vi "plcHMI_rev6.vi"() -> ()   [LabVIEW 2020]
doc: "ADS continuos synchronous write example using base blocks. \n\nThe client writes data synchronously and does wait for the respose from server."
uses:
  Agilent/AgilentTotalCluster.ctl
  Agilent/AgilentControl.ctl
  Agilent/Channel Config.ctl
  <vilib>/Platform/TimedLoop/XDataNode/timing_clust.ctl
  <vilib>/Platform/TimedLoop/XDataNode/nitl_modes.ctl
  <vilib>/Platform/TimedLoop/XDataNode/wakeup.ctl
  <userlib>/Beckhoff-LabVIEW-Interface/_DependsOn/With TypeResolving/Write Sync Single TypeResolved.vi
  <userlib>/Beckhoff-LabVIEW-Interface/_DependsOn/With TypeResolving/Read Sync Single TypeResolved.vi
  <vilib>/Platform/TimedLoop/XDataNode/XDataNode.xnode
  <vilib>/Platform/TimedLoop/XDataNode/XDNodeRunTimeDep.lvlib
panel:
  in  "Tab Control":T1(tab)
  out "error out":errorcluster
  in  "Symbol file path - MUST BE ENTERED\nLoad \"ADS Write AND Read Symbols REV X.X.xml\"":path
  out "bHasMached":bool
  out "Write Status":bool
  out "Read Status":bool
  in  "EXIT HMI":bool caption="STOP HMI\nEXIT HMI"
  out "Internal TwinCAT Handle ID Maps":dbl format="%#_12g"
  in  "802L TDK PSU Voltage Rating (abs(Volts))":i32=12000 min=1 max=50000
  in  "802L TDL PSU Peak Power (J/s)":i32=9000 min=1 max=50000
  in  "HVPS Model":u16(ring) items=["802L-12kV,9000J/s", "802L+50kV,9000J/s", "Other"]
  out "Test Interval Fault":bool
  in  "Cycle Time (Sec)":i32=15 min=0
  in  "Voltage Held by PSU":bool
  in  "Log Capacitor Voltage":bool
  in  "Log Temperature Data":bool
  out "Time Since Last Shot":string caption="Elapsed Time Text"
  in  "Duty Cycle":dbl
  in  "Current Control":bool
  out "Expected Voltage":i16
  in  "Dump":bool
  out "EOC":bool
  out "Maximum Test Number Reached":bool
  out "SCR Ready":bool
  in  "START":bool
  in  "STOP":bool
  in  "Hold":bool
  in  "Charge":bool
  in  "Shot":bool
  in  "HV Switch Mode":bool
  in  "CLEAR FAULT":bool
  in  "Manual/Auto":bool=TRUE
  out "Test Interval (Sec)":i32=15 min=0
  in  "Capacitance (uF)":sgl=1e-13 min=0 max=10000 format="%#_6f"
  in  "Target Charge Volt (V) - Min 1500V":i32 min=-12000 max=50000 step=1
  out "Estimated Charge Time (seconds)":sgl
  in  "Hold Time Before Shot (seconds)":sgl max=1000
  in  "Max Number of Shots (Test intervals)":i16=1 min=1
  out "Shot Number":i16
  out "Charge Fault":bool=TRUE
  out "Discharge Fault":bool=TRUE
  out "Hold Fault":bool=TRUE
  out "Cap 1 Temp\nExceeded Fault":bool=TRUE
  out "Ambient Temp\nExceeded Fault":bool=TRUE
  out "PSU Fault":bool=TRUE
  out "Control Sys Fault":bool=TRUE
  out "test Running":bool
  out "Test State":string
  out "Cap 1 Voltage":i16
  out "Cap 1 Temperature":i16
  in  "Capacitor Voltage Data Log File Path (.xlsx)":path
  out "Load Temperature":i16
  out "Soft Dump Temp":i16
  out "Ambient Temp":i16
  out "Waveform Chart - Capacitor Voltage (Probe, abs(Volts))":dbl(graph)
  in  "Manual Charge Time (seconds)":sgl max=90
  in  "Reset Test Number":bool
  in  "Cap 1 Fault Temp (Cel)":i16 min=0 max=300
  in  "Capacitor Temperature Data Log File Path (.xlsx)":path
  out "Cap 1 Voltage (HVPS)":i16
  in  "50kV PSU Charger Selected\n(OFF = 12kV Selected, ON = 50kV) Selected":bool
  in  "Cap Rated Voltage (V)":u16 max=50000
  out "Target Voltage Exceeded\nCap Rating Voltage":bool=TRUE
  in  "Soft Dump Temp Thres (Cel)":i16 min=0 max=500
  in  "Load Temp Thres (Cel)":i16 min=0 max=500
  in  "Ambient Temp Thres (Cel)":i16 min=0 max=500
  out "All Temp In Range":bool=TRUE
  out "Load Temp Fault":bool=TRUE
  out "Capacitor Voltage":cluster{dbl, dbl}(graph)
  out "EOC":i16(graph)
  out "Soft Exception":bool
  out "PSU HV FB Fault":bool
  out "Charge FB Fault":bool
  out "Softdump FB Fault":bool
  out "SCR FB":i16(graph)
  out "Spark Gap Voltage":i16(graph)
  in  "CH4 Vertical Units":string(combo)="V"
  in  "CH4 Vertical Units/div":dbl=2.0
  in  "Toggle Scope Scale":bool
  in  "CH1 Vertical Units/div":dbl=2.0
  in  "CH1 Vertical Units":string(combo)="V"
  in  "Horizontal Units":enum16{"us", "ms", "s"}(ring)
  in  "Horizontal Units/div":dbl=200.0
  out "Download":bool
  in  "Single":bool
  in  "Stop":bool
  out "Scope Trig":bool
  in  "Agilent Array":T2[](array[typedef])
  out "Process Step":u8
  out "Stop Loops":bool
  # "CONFIGURATION"
  # "Press STOP HMI instead of\nLabView Abort Execution"
  # "PSU V Rating, Peak Power\nactive when OTHER\nis selected"
  # "INPUT VARIABLES - For TDK Lambda 802L\nMust be written to before START"
  # "FAULT STATUSES"
  # "Set to -1 for automated\nfull charge to setpoint"
  # "MANUAL CONTROLS"
  # "Does not record during \"wait\" and appends to data file. Must be named with .xlsx"
  # "HV Switch Configuration"
  # "Records during \"Test Running.\" Must be named with .xlsx"
  # "Control Sys Faults"
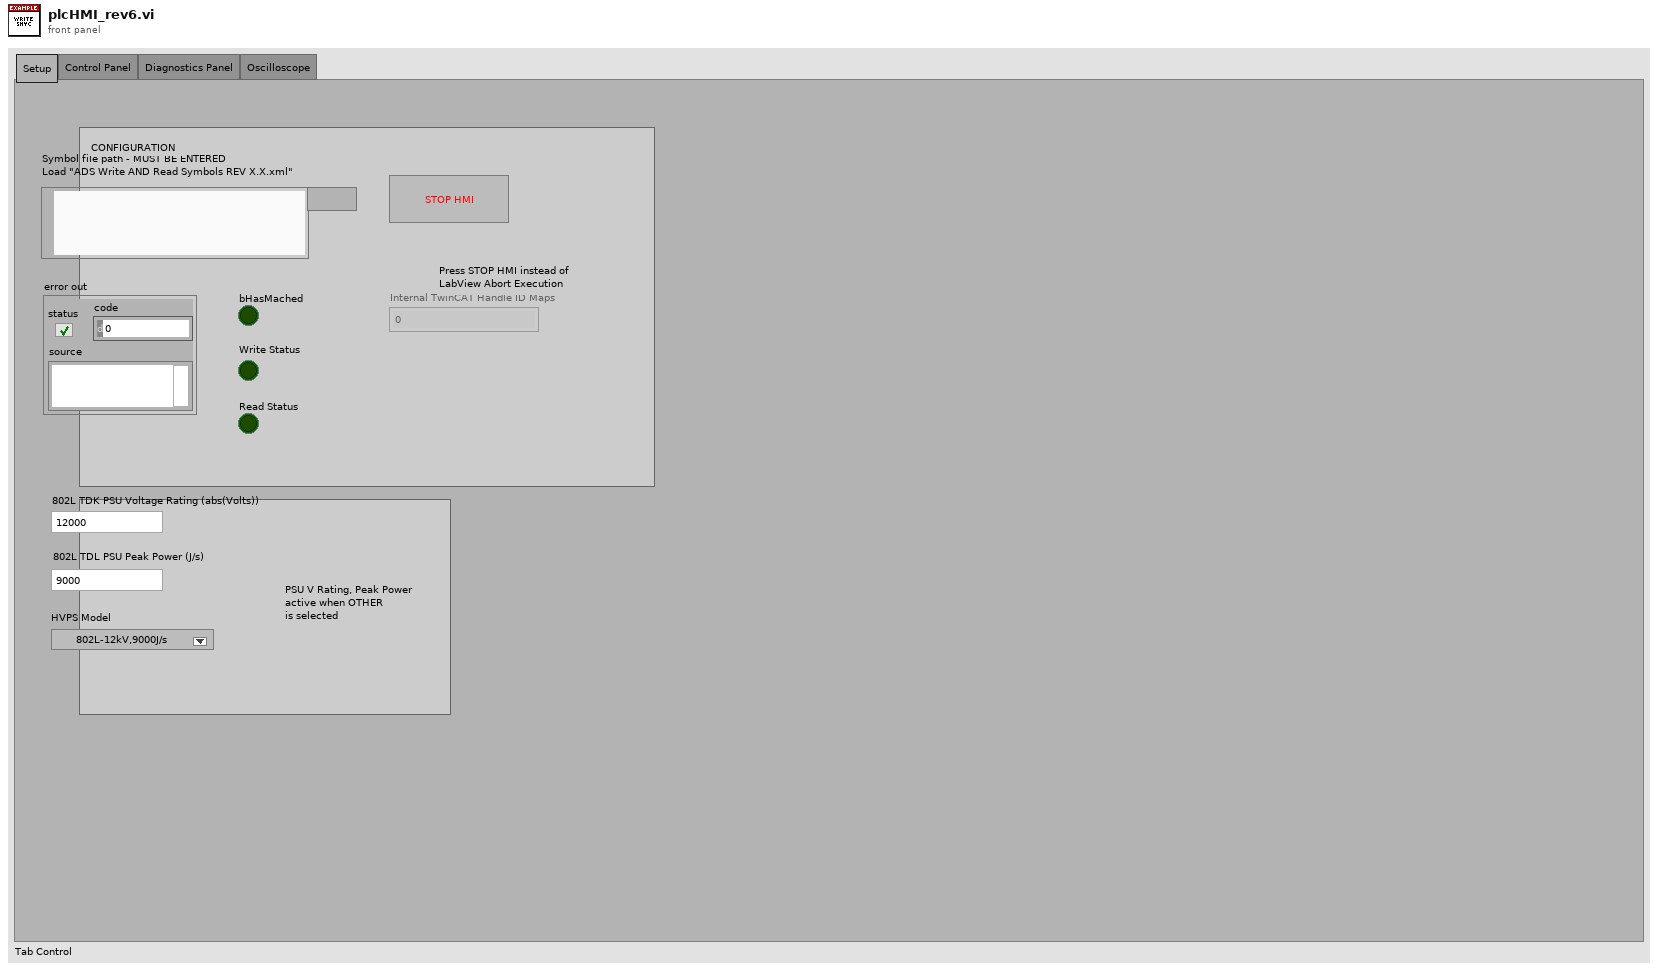
[diagram p1: front panel]
types:
  T1 = enum32{"Setup", "Control Panel", "Diagnostics Panel", "Oscilloscope"}
  T2 = typedef "AgilentTotalCluster.ctl" = cluster{"Agilent Graph":waveform(dbl)[], "Agilent Control":T3, "Agilent Setup Error":errorcluster, "Agilent Present":bool, "Enabled":bool}
  T3 = typedef "AgilentControl.ctl" = cluster{"Trig?":bool, "VISA session":refnum<visa-resource-name>, "Setup to Load":string, "Timeout (ms)":u32, "Desired Samp":enum32{"100", "250", "500", "1000", "2000", "5000", "10000", "20000", "50000", "100000", "200000", "500000", "1000000", "2000000", "4000000", "8000000"}, "Captured Samp":i32, "Desired Channels":T4[]}
  T4 = typedef "Channel Config.ctl" = cluster{"Chan Index":enum16{"Channel1", "Channel2", "Channel3", "Channel4", "MATH"}, "Name":string, "Samples":i32}
  T5 = typedef "XDNodeRunTimeDep.lvlib/timing_clust.ctl" = cluster{"Expected End [f-1]":u64, "Actual End [f-1]":u64, "Finished Late? [f-1]":bool, "Expected End [i-1]":u64, "Actual End [i-1]":u64, "Finished Late? [i-1]":bool, "Expected Start [i]":u64, "Actual Start [i]":u64, "Expected Start [f]":u64, "Actual Start [f]":u64, "Source Name":string, "Structure Name":string, "Period":i64, "Deadline":i64, "Offset":i64, "Start":i64, "Priority":i32, "Timeout":i32, "Mode":T6, "Wakeup Reason":T7, "Error":errorcluster, "Source Type":string, "Secondary Source Type":string, "Global End Time":u64, "Global Start Time":u64, "Frame Duration":u64, "Iteration Duration":u64, "Assigned CPU":i32, "I/O Scan Engine Mode":u32}
  T6 = typedef "XDNodeRunTimeDep.lvlib/nitl_modes.ctl" = enum32{"No Change", "Process missed periods, maintain original phase", "Discard missed periods, maintain original phase", "Process missed periods, ignore original phase", "Discard missed periods, ignore original phase"}
  T7 = typedef "XDNodeRunTimeDep.lvlib/wakeup.ctl" = enum32{"Normal", "Aborted", "Asynchronous wakeup", "Timing source error", "Timed loop error", "Timeout"}
  T8 = cluster{"Agilent Array[0]":T2, "Agilent Array[1]":T2, "Agilent Array[2]":T2, "Agilent Array[3]":T2, "Agilent Array[4]":T2, "Agilent Array[5]":T2, "Agilent Array[6]":T2, "Agilent Array[7]":T2, "Agilent Array[8]":T2}
  T9 = enum32{"100", "250", "500", "1000", "2000", "5000", "10000", "20000", "50000", "100000", "200000", "500000", "1000000", "2000000", "4000000", "8000000"}
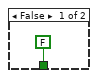
[diagram p2: hidden frame]
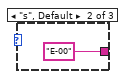
[diagram p5: hidden frame]
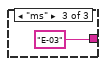
[diagram p6: hidden frame]
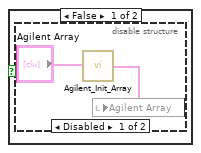
[diagram p7: hidden frame]
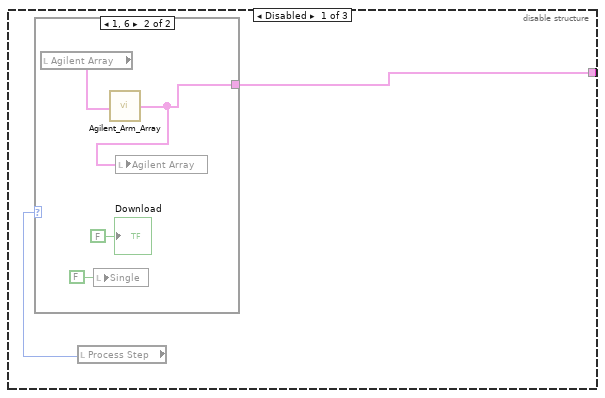
[diagram p11: hidden frame]
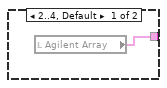
[diagram p12: hidden frame]
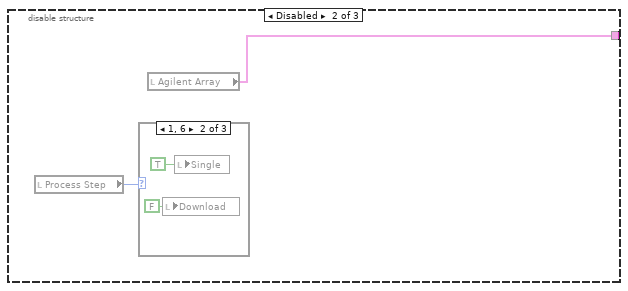
[diagram p13: hidden frame]
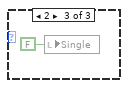
[diagram p15: hidden frame]
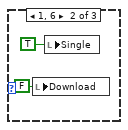
[diagram p17: hidden frame]
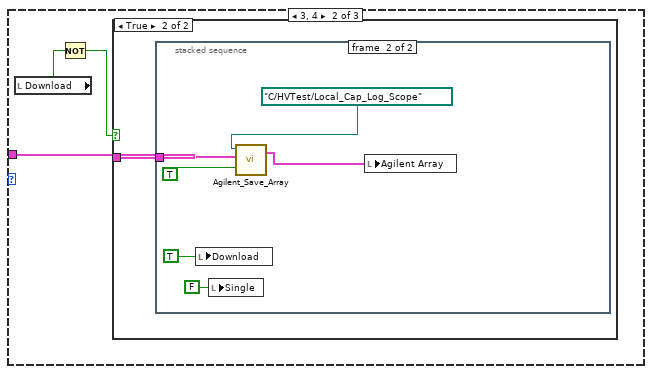
[diagram p19: hidden frame]
diagram:
  w115 = u16 17 items=["SyncLatest"=17, "AsyncLatest"=33] ("WriterMode")
  w185 = u16 33 items=["SyncLatest"=17, "AsyncLatest"=33] ("WriterMode")
  w225 = u16 33 items=["SyncLatest"=17, "AsyncLatest"=33] ("WriterMode")
  w244 = u16 33 items=["SyncLatest"=17, "AsyncLatest"=33] ("WriterMode")
  w263 = u16 33 items=["SyncLatest"=17, "AsyncLatest"=33] ("WriterMode")
  w282 = u16 33 items=["SyncLatest"=17, "AsyncLatest"=33] ("WriterMode")
  w301 = u16 33 items=["SyncLatest"=17, "AsyncLatest"=33] ("WriterMode")
  w320 = u16 17 items=["SyncLatest"=17, "AsyncLatest"=33] ("WriterMode")
  w339 = u16 17 items=["SyncLatest"=17, "AsyncLatest"=33] ("WriterMode")
  w358 = u16 17 items=["SyncLatest"=17, "AsyncLatest"=33] ("WriterMode")
  w377 = u16 17 items=["SyncLatest"=17, "AsyncLatest"=33] ("WriterMode")
  w396 = u16 17 items=["SyncLatest"=17, "AsyncLatest"=33] ("WriterMode")
  w415 = u16 17 items=["SyncLatest"=17, "AsyncLatest"=33] ("WriterMode")
  w434 = u16 17 items=["SyncLatest"=17, "AsyncLatest"=33] ("WriterMode")
  w449 = u16 17 items=["SyncLatest"=17, "AsyncLatest"=33] ("WriterMode")
  # "Variables/ Control"
  # "Documentation:\nCode separated vertically into two main sections - Write and read\nThey are further separated into BOOL and numeric\nThe OR gates wire all the error lines and the EXIT HMI button to a WHILE LOOP STOP\nThere current delay time on the routine is 100ms\nAll the AND gates connect the typecast resolve lines to the bHasMatched indicator\nThe second and third set of AND gates connect the write statuses to the Write Status indicator\nThe same is done for the read status indicator"
  # "WRITE NUMERICS"
  # "WRITE BOOLS"
  # "Select Symbol N"
  # "Read Initialization"
  # "Release \nTypeResolver"
  # "Release Writer"
  # "Send Request"
  # "Init \nTypeResolver"
  # "Init Writer"
  # "Select Symbol"
  # "Initialization"
  # "Call Release handle block\nat the end, when all nodes\nhave finished their execution"
  # "There must be only one release\nafter every init block.\nRelease block must be called\nalways at the end."
  # "Release"
  # "Symbol Interface"
  n1 = disable-structure shown="Enabled" {
    disable-tunnel: [w455 _] -> w453
    disable-tunnel: [w454 w457] -> w452
    frame Disabled {
      # "Using Symbol Interface"
      n2 = call <userlib>:"Symbol Interface.vi"() -> ("PortInfo"=w454:string, "error out"=w455:errorcluster)  [unwired: 14 in]
    }
    frame Enabled {
      # "Using Symbol File"
      n3 = Path To String(path="Symbol file path - MUST BE ENTERED\nLoad \"ADS Write AND Read Symbols REV X.X.xml\"") -> (string=w457:string)
    }
  }
  n4 = call <userlib>:"Init.vi"("XMLDescription"=w452, "error in (no error)"=w453) -> ("Handle"=w65:u32, "ReadGrpSymbols"=w5:string[], "WriteGrpSymbols"=w10:string[], "error out"=w32:errorcluster)  [unwired: 9 in, 1 out]
  n5 = Index Array(array=w10, index=0) -> (element=w43:string)
  n6 = Index Array(array=w10, index=26) -> (element=w9:string)
  n7 = Index Array(array=w10, index=24) -> (element=w16:string)
  n8 = Index Array(array=w10, index=23) -> (element=w22:string)
  n9 = Index Array(array=w10, index=22) -> (element=w25:string)
  n10 = Index Array(array=w10, index=25) -> (element=w13:string)
  n11 = Index Array(array=w10, index=21) -> (element=w53:string)
  n12 = Index Array(array=w10, index=20) -> (element=w58:string)
  n13 = Index Array(array=w10, index=14) -> (element=w33:string)
  n14 = Index Array(array=w10, index=9) -> (element=w302:string)
  n15 = Index Array(array=w10, index=10) -> (element=w283:string)
  n16 = Index Array(array=w10, index=12) -> (element=w245:string)
  n17 = Index Array(array=w10, index=11) -> (element=w264:string)
  n18 = Index Array(array=w10, index=13) -> (element=w226:string)
  n19 = Index Array(array=w10, index=18) -> (element=w66:string)
  n20 = Index Array(array=w10, index=19) -> (element=w59:string)
  n21 = Index Array(array=w10, index=7) -> (element=w321:string)
  n22 = Index Array(array=w10, index=2) -> (element=w416:string)
  n23 = Index Array(array=w10, index=3) -> (element=w397:string)
  n24 = Index Array(array=w10, index=5) -> (element=w359:string)
  n25 = Index Array(array=w10, index=4) -> (element=w378:string)
  n26 = Index Array(array=w10, index=6) -> (element=w340:string)
  n27 = Index Array(array=w10, index=1) -> (element=w435:string)
  n28 = Index Array(array=w10, index=16) -> (element=w36:string)
  n29 = Index Array(array=w10, index=8) -> (element=w114:string)
  n30 = Index Array(array=w10, index=15) -> (element=w186:string)
  n31 = Index Array(array=w10, index=17) -> (element=w38:string)
  n32 = call <userlib>:"Init Writer.vi"("Handle"=w65, "SymbolName"=w302, "WriterMode"=w301, "error constant"=w32) -> ("Handle"=w297:u32, "SymbolName"=w296:string, "WriterMode"=w295:u16, "WriteHandle"=w293:u32, "error IO"=w294:errorcluster)  [unwired: 7 in]
  n33 = call <userlib>:"Init Writer.vi"("Handle"=w65, "SymbolName"=w283, "WriterMode"=w282, "error constant"=w32) -> ("Handle"=w281:u32, "SymbolName"=w280:string, "WriterMode"=w279:u16, "WriteHandle"=w278:u32, "error IO"=w277:errorcluster)  [unwired: 7 in]
  n34 = call <userlib>:"Init Writer.vi"("Handle"=w65, "SymbolName"=w245, "WriterMode"=w244, "error constant"=w32) -> ("Handle"=w243:u32, "SymbolName"=w242:string, "WriterMode"=w241:u16, "WriteHandle"=w240:u32, "error IO"=w239:errorcluster)  [unwired: 7 in]
  n35 = call <userlib>:"Init Type.vi"("Handle"=w65, "SymbolName"=w302, "error in"=w32) -> ("Handle"=w286:u32, "TypeHdl"=w285:u32, "error IO"=w284:errorcluster)  [unwired: 7 in, 3 out]
  n36 = call <userlib>:"Init Type.vi"("Handle"=w65, "SymbolName"=w283, "error in"=w32) -> ("Handle"=w276:u32, "TypeHdl"=w275:u32, "error IO"=w274:errorcluster)  [unwired: 7 in, 3 out]
  n37 = call <userlib>:"Init Writer.vi"("Handle"=w65, "SymbolName"=w264, "WriterMode"=w263, "error constant"=w32) -> ("Handle"=w262:u32, "SymbolName"=w261:string, "WriterMode"=w260:u16, "WriteHandle"=w259:u32, "error IO"=w258:errorcluster)  [unwired: 7 in]
  n38 = call <userlib>:"Init Type.vi"("Handle"=w65, "SymbolName"=w245, "error in"=w32) -> ("Handle"=w238:u32, "TypeHdl"=w237:u32, "error IO"=w236:errorcluster)  [unwired: 7 in, 3 out]
  n39 = call <userlib>:"Init Writer.vi"("Handle"=w65, "SymbolName"=w226, "WriterMode"=w225, "error constant"=w32) -> ("Handle"=w224:u32, "SymbolName"=w223:string, "WriterMode"=w222:u16, "WriteHandle"=w221:u32, "error IO"=w220:errorcluster)  [unwired: 7 in]
  n40 = call <userlib>:"Init Type.vi"("Handle"=w65, "SymbolName"=w264, "error in"=w32) -> ("Handle"=w257:u32, "TypeHdl"=w256:u32, "error IO"=w255:errorcluster)  [unwired: 7 in, 3 out]
  n41 = call <userlib>:"Init Type.vi"("Handle"=w65, "SymbolName"=w226, "error in"=w32) -> ("Handle"=w219:u32, "TypeHdl"=w218:u32, "error IO"=w217:errorcluster)  [unwired: 7 in, 3 out]
  n42 = Index Array(array=w5, index=21) -> (element=w80:string)
  n43 = Index Array(array=w5, index=22) -> (element=w77:string)
  n44 = call <userlib>:"Init Writer.vi"("Handle"=w65, "SymbolName"=w321, "WriterMode"=w320, "error constant"=w32) -> ("Handle"=w319:u32, "SymbolName"=w318:string, "WriterMode"=w317:u16, "WriteHandle"=w316:u32, "error IO"=w315:errorcluster)  [unwired: 7 in]
  n45 = Index Array(array=w5, index=20) -> (element=w85:string)
  n46 = call <userlib>:"Init Writer.vi"("Handle"=w65, "SymbolName"=w416, "WriterMode"=w415, "error constant"=w32) -> ("Handle"=w411:u32, "SymbolName"=w410:string, "WriterMode"=w409:u16, "WriteHandle"=w407:u32, "error IO"=w408:errorcluster)  [unwired: 7 in]
  n47 = call <userlib>:"Init Writer.vi"("Handle"=w65, "SymbolName"=w397, "WriterMode"=w396, "error constant"=w32) -> ("Handle"=w395:u32, "SymbolName"=w394:string, "WriterMode"=w393:u16, "WriteHandle"=w392:u32, "error IO"=w391:errorcluster)  [unwired: 7 in]
  n48 = call <userlib>:"Init Writer.vi"("Handle"=w65, "SymbolName"=w359, "WriterMode"=w358, "error constant"=w32) -> ("Handle"=w357:u32, "SymbolName"=w356:string, "WriterMode"=w355:u16, "WriteHandle"=w354:u32, "error IO"=w353:errorcluster)  [unwired: 7 in]
  n49 = call <userlib>:"Init Type.vi"("Handle"=w65, "SymbolName"=w321, "error in"=w32) -> ("Handle"=w314:u32, "TypeHdl"=w313:u32, "error IO"=w312:errorcluster)  [unwired: 7 in, 3 out]
  n50 = Index Array(array=w5, index=23) -> (element=w76:string)
  n51 = call <userlib>:"Init Type.vi"("Handle"=w65, "SymbolName"=w416, "error in"=w32) -> ("Handle"=w400:u32, "TypeHdl"=w399:u32, "error IO"=w398:errorcluster)  [unwired: 7 in, 3 out]
  n52 = call <userlib>:"Init Type.vi"("Handle"=w65, "SymbolName"=w397, "error in"=w32) -> ("Handle"=w390:u32, "TypeHdl"=w389:u32, "error IO"=w388:errorcluster)  [unwired: 7 in, 3 out]
  n53 = call <userlib>:"Init Writer.vi"("Handle"=w65, "SymbolName"=w378, "WriterMode"=w377, "error constant"=w32) -> ("Handle"=w376:u32, "SymbolName"=w375:string, "WriterMode"=w374:u16, "WriteHandle"=w373:u32, "error IO"=w372:errorcluster)  [unwired: 7 in]
  n54 = call <userlib>:"Init Type.vi"("Handle"=w65, "SymbolName"=w359, "error in"=w32) -> ("Handle"=w352:u32, "TypeHdl"=w351:u32, "error IO"=w350:errorcluster)  [unwired: 7 in, 3 out]
  n55 = call <userlib>:"Init Writer.vi"("Handle"=w65, "SymbolName"=w340, "WriterMode"=w339, "error constant"=w32) -> ("Handle"=w338:u32, "SymbolName"=w337:string, "WriterMode"=w336:u16, "WriteHandle"=w335:u32, "error IO"=w334:errorcluster)  [unwired: 7 in]
  n56 = Index Array(array=w5, index=16) -> (element=w169:string)
  n57 = Index Array(array=w5, index=24) -> (element=w74:string)
  n58 = Index Array(array=w5, index=28) -> (element=w29:string)
  n59 = Index Array(array=w5, index=30) -> (element=w4:string)
  n60 = call <userlib>:"Init Type.vi"("Handle"=w65, "SymbolName"=w378, "error in"=w32) -> ("Handle"=w371:u32, "TypeHdl"=w370:u32, "error IO"=w369:errorcluster)  [unwired: 7 in, 3 out]
  n61 = call <userlib>:"Init Type.vi"("Handle"=w65, "SymbolName"=w340, "error in"=w32) -> ("Handle"=w333:u32, "TypeHdl"=w332:u32, "error IO"=w331:errorcluster)  [unwired: 7 in, 3 out]
  n62 = call <userlib>:"Init Writer.vi"("Handle"=w65, "SymbolName"=w435, "WriterMode"=w434, "error constant"=w32) -> ("Handle"=w433:u32, "SymbolName"=w432:string, "WriterMode"=w431:u16, "WriteHandle"=w430:u32, "error IO"=w429:errorcluster)  [unwired: 7 in]
  n63 = Index Array(array=w5, index=11) -> (element=w191:string)
  n64 = call <userlib>:"Init Type.vi"("Handle"=w65, "SymbolName"=w435, "error in"=w32) -> ("Handle"=w428:u32, "TypeHdl"=w427:u32, "error IO"=w426:errorcluster)  [unwired: 7 in, 3 out]
  n65 = Index Array(array=w5, index=10) -> (element=w192:string)
  n66 = Index Array(array=w5, index=17) -> (element=w88:string)
  n67 = Index Array(array=w5, index=18) -> (element=w87:string)
  n68 = call <userlib>:"Init Writer.vi"("Handle"=w65, "SymbolName"=w43, "WriterMode"=w449, "error constant"=w32) -> ("Handle"=w448:u32, "SymbolName"=w447:string, "WriterMode"=w446:u16, "WriteHandle"=w445:u32, "error IO"=w444:errorcluster)  [unwired: 7 in]
  n69 = Index Array(array=w5, index=29) -> (element=w19:string)
  n70 = call <userlib>:"Init Type.vi"("Handle"=w65, "SymbolName"=w43, "error in"=w32) -> ("Handle"=w443:u32, "TypeHdl"=w442:u32, "error IO"=w437:errorcluster)  [unwired: 7 in, 3 out]
  n71 = call <userlib>:"Init Writer.vi"("Handle"=w65, "SymbolName"=w186, "WriterMode"=w185, "error constant"=w32) -> ("Handle"=w181:u32, "SymbolName"=w180:string, "WriterMode"=w179:u16, "WriteHandle"=w171:u32, "error IO"=w178:errorcluster)  [unwired: 7 in]
  n72 = Index Array(array=w5, index=13) -> (element=w189:string)
  n73 = Index Array(array=w5, index=27) -> (element=w47:string)
  n74 = call <userlib>:"Init Type.vi"("Handle"=w65, "SymbolName"=w186, "error in"=w32) -> ("Handle"=w176:u32, "TypeHdl"=w174:u32, "error IO"=w175:errorcluster)  [unwired: 7 in, 3 out]
  n75 = Index Array(array=w5, index=12) -> (element=w190:string)
  n76 = Index Array(array=w5, index=15) -> (element=w187:string)
  n77 = Index Array(array=w5, index=19) -> (element=w86:string)
  n78 = Index Array(array=w5, index=26) -> (element=w48:string)
  n79 = Index Array(array=w5, index=5) -> (element=w99:string)
  n80 = Index Array(array=w5, index=6) -> (element=w157:string)
  n81 = Index Array(array=w5, index=9) -> (element=w201:string)
  n82 = Index Array(array=w5, index=14) -> (element=w188:string)
  n83 = Index Array(array=w5, index=8) -> (element=w159:string)
  n84 = Index Array(array=w5, index=25) -> (element=w63:string)
  n85 = Index Array(array=w5, index=31) -> (element=w3:string)
  n86 = call <userlib>:"Init Writer.vi"("Handle"=w65, "SymbolName"=w114, "WriterMode"=w115, "error constant"=w32) -> ("Handle"=w113:u32, "SymbolName"=w112:string, "WriterMode"=w111:u16, "WriteHandle"=w110:u32, "error IO"=w109:errorcluster)  [unwired: 7 in]
  n87 = Index Array(array=w5, index=7) -> (element=w158:string)
  n88 = call <userlib>:"Init Type.vi"("Handle"=w65, "SymbolName"=w114, "error in"=w32) -> ("Handle"=w108:u32, "TypeHdl"=w107:u32, "error IO"=w106:errorcluster)  [unwired: 7 in, 3 out]
  n89 = Index Array(array=w5, index=2) -> (element=w167:string)
  n90 = Index Array(array=w5, index=4) -> (element=w163:string)
  n91 = Index Array(array=w5, index=0) -> (element=w202:string)
  n92 = Index Array(array=w5, index=1) -> (element=w203:string)
  n93 = Index Array(array=w5, index=3) -> (element=w164:string)
  n94 = node-c288(i64 10 ("Period")) -> (w123:T5)  [unwired: 2 in]
  n95 = timed-loop {
    tunnel: w448 -> [w815]
    tunnel: w447 -> [w814]
    tunnel: w446 -> [w813]
    tunnel: w445 -> [w812]
    tunnel: w443 -> [w1057]
    tunnel: w442 -> [w1056]
    tunnel: [w810] -> w441
    tunnel: [w809] -> w440
    tunnel: [w1055] -> w439
    tunnel: [w1054] -> w438
    tunnel: w433 -> [w1052]
    tunnel: w432 -> [w1051]
    tunnel: w431 -> [w1050]
    tunnel: w430 -> [w1049]
    tunnel: w428 -> [w1047]
    tunnel: w427 -> [w1046]
    tunnel: [w1044] -> w424
    tunnel: [w1043] -> w423
    tunnel: [w1042] -> w421
    tunnel: [w1041] -> w420
    tunnel: w411 -> [w1040]
    tunnel: w410 -> [w1039]
    tunnel: w409 -> [w1038]
    tunnel: w407 -> [w1036]
    tunnel: [w1035] -> w406
    tunnel: [w1034] -> w405
    tunnel: [w1033] -> w402
    tunnel: [w1032] -> w401
    tunnel: w400 -> [w1031]
    tunnel: w399 -> [w1030]
    tunnel: w395 -> [w1028]
    tunnel: w394 -> [w1027]
    tunnel: w393 -> [w1026]
    tunnel: w392 -> [w1025]
    tunnel: w390 -> [w1023]
    tunnel: w389 -> [w1022]
    tunnel: [w1020] -> w386
    tunnel: [w1019] -> w385
    tunnel: [w1018] -> w383
    tunnel: [w1017] -> w382
    tunnel: w376 -> [w1016]
    tunnel: w375 -> [w1015]
    tunnel: w374 -> [w1014]
    tunnel: w373 -> [w1013]
    tunnel: w371 -> [w1011]
    tunnel: w370 -> [w1010]
    tunnel: [w1008] -> w367
    tunnel: [w1007] -> w366
    tunnel: [w1006] -> w364
    tunnel: [w1005] -> w363
    tunnel: w357 -> [w1004]
    tunnel: w356 -> [w1003]
    tunnel: w355 -> [w1002]
    tunnel: w354 -> [w1001]
    tunnel: w352 -> [w999]
    tunnel: w351 -> [w998]
    tunnel: [w996] -> w348
    tunnel: [w995] -> w347
    tunnel: [w994] -> w345
    tunnel: [w993] -> w344
    tunnel: w338 -> [w992]
    tunnel: w337 -> [w991]
    tunnel: w336 -> [w990]
    tunnel: w335 -> [w989]
    tunnel: w333 -> [w987]
    tunnel: w332 -> [w986]
    tunnel: [w984] -> w329
    tunnel: [w983] -> w328
    tunnel: [w982] -> w326
    tunnel: [w981] -> w325
    tunnel: w319 -> [w980]
    tunnel: w318 -> [w979]
    tunnel: w317 -> [w978]
    tunnel: w316 -> [w977]
    tunnel: w314 -> [w975]
    tunnel: w313 -> [w974]
    tunnel: [w972] -> w310
    tunnel: [w971] -> w309
    tunnel: [w970] -> w307
    tunnel: [w969] -> w306
    tunnel: w297 -> [w968]
    tunnel: w296 -> [w967]
    tunnel: w295 -> [w966]
    tunnel: w293 -> [w964]
    tunnel: [w963] -> w292
    tunnel: [w962] -> w291
    tunnel: [w961] -> w288
    tunnel: [w960] -> w287
    tunnel: w286 -> [w959]
    tunnel: w285 -> [w958]
    tunnel: w281 -> [w956]
    tunnel: w280 -> [w955]
    tunnel: w279 -> [w954]
    tunnel: w278 -> [w953]
    tunnel: w276 -> [w951]
    tunnel: w275 -> [w950]
    tunnel: [w948] -> w272
    tunnel: [w947] -> w271
    tunnel: [w946] -> w269
    tunnel: [w945] -> w268
    tunnel: w262 -> [w944]
    tunnel: w261 -> [w943]
    tunnel: w260 -> [w942]
    tunnel: w259 -> [w941]
    tunnel: w257 -> [w939]
    tunnel: w256 -> [w938]
    tunnel: [w936] -> w253
    tunnel: [w935] -> w252
    tunnel: [w934] -> w250
    tunnel: [w933] -> w249
    tunnel: w243 -> [w932]
    tunnel: w242 -> [w931]
    tunnel: w241 -> [w930]
    tunnel: w240 -> [w929]
    tunnel: w238 -> [w927]
    tunnel: w237 -> [w926]
    tunnel: [w924] -> w234
    tunnel: [w923] -> w233
    tunnel: [w922] -> w231
    tunnel: [w921] -> w230
    tunnel: w224 -> [w920]
    tunnel: w223 -> [w919]
    tunnel: w222 -> [w918]
    tunnel: w221 -> [w917]
    tunnel: w219 -> [w915]
    tunnel: w218 -> [w914]
    tunnel: [w912] -> w215
    tunnel: [w911] -> w214
    tunnel: [w910] -> w212
    tunnel: [w909] -> w211
    tunnel: w203 -> [w908]
    tunnel: w202 -> [w907]
    tunnel: w201 -> [w906]
    tunnel: [w905] -> w152
    tunnel: w192 -> [w904]
    tunnel: w191 -> [w903]
    tunnel: w190 -> [w902]
    tunnel: w189 -> [w901]
    tunnel: w188 -> [w900]
    tunnel: w187 -> [w899]
    tunnel: [w898] -> w120
    tunnel: [w897] -> w151
    tunnel: [w896] -> w150
    tunnel: [w895] -> w149
    tunnel: [w894] -> w148
    tunnel: [w838] -> w147
    tunnel: [w836] -> w146
    shift-right: [w739] -> w451
    shift-left: w444 -> [w811]
    shift-right: [w738] -> w450
    shift-left: w437 -> [w1053]
    shift-right: [w736] -> w422
    shift-left: w429 -> [w1048]
    shift-right: [w735] -> w419
    shift-left: w426 -> [w1045]
    shift-right: [w733] -> w404
    shift-left: w408 -> [w1037]
    shift-right: [w732] -> w403
    shift-left: w398 -> [w1029]
    shift-right: [w730] -> w384
    shift-left: w391 -> [w1024]
    shift-right: [w729] -> w381
    shift-left: w388 -> [w1021]
    shift-right: [w727] -> w365
    shift-left: w372 -> [w1012]
    shift-right: [w726] -> w362
    shift-left: w369 -> [w1009]
    shift-right: [w724] -> w346
    shift-left: w353 -> [w1000]
    shift-right: [w723] -> w343
    shift-left: w350 -> [w997]
    shift-right: [w721] -> w327
    shift-left: w334 -> [w988]
    shift-right: [w720] -> w324
    shift-left: w331 -> [w985]
    shift-right: [w718] -> w308
    shift-left: w315 -> [w976]
    shift-right: [w717] -> w305
    shift-left: w312 -> [w973]
    shift-right: [w716] -> w290
    shift-left: w294 -> [w965]
    shift-right: [w715] -> w289
    shift-left: w284 -> [w957]
    shift-right: [w713] -> w270
    shift-left: w277 -> [w952]
    shift-right: [w712] -> w267
    shift-left: w274 -> [w949]
    shift-right: [w710] -> w251
    shift-left: w258 -> [w940]
    shift-right: [w709] -> w248
    shift-left: w255 -> [w937]
    shift-right: [w707] -> w232
    shift-left: w239 -> [w928]
    shift-right: [w706] -> w229
    shift-left: w236 -> [w925]
    shift-right: [w704] -> w213
    shift-left: w220 -> [w916]
    shift-right: [w703] -> w210
    shift-left: w217 -> [w913]
    tunnel: w181 -> [w878]
    tunnel: w180 -> [w877]
    tunnel: w179 -> [w876]
    tunnel: [w874] -> w42
    tunnel: [w873] -> w177
    tunnel: w176 -> [w872]
    tunnel: w174 -> [w870]
    tunnel: [w869] -> w173
    tunnel: [w868] -> w172
    tunnel: w171 -> [w867]
    tunnel: w169 -> [w866]
    tunnel: [w837] -> w145
    tunnel: [w860] -> w154
    tunnel: w32 -> [w859]
    tunnel: [w857] -> w153
    tunnel: w167 -> [w856]
    tunnel: w164 -> [w852]
    tunnel: w163 -> [w851]
    tunnel: [w842] -> w155
    tunnel: [w841] -> w156
    tunnel: w159 -> [w835]
    tunnel: w158 -> [w834]
    tunnel: w157 -> [w833]
    tunnel: [w820] -> w96
    tunnel: [w819] -> w95
    tunnel: [w818] -> w94
    timing: w123 -> [_]
    timing-out: [_] -> w122
    tunnel: w65 -> [w808]
    tunnel: [w701] -> w98
    tunnel: w113 -> [w696]
    tunnel: w112 -> [w695]
    tunnel: w111 -> [w694]
    tunnel: w110 -> [w693]
    tunnel: w108 -> [w691]
    tunnel: w107 -> [w690]
    tunnel: [w687] -> w105
    tunnel: [w686] -> w104
    tunnel: [w685] -> w103
    tunnel: [w684] -> w102
    tunnel: [w677] -> w97
    tunnel: w99 -> [w673]
    tunnel: [w672] -> w93
    tunnel: w88 -> [w668]
    tunnel: w87 -> [w663]
    tunnel: w86 -> [w662]
    tunnel: w85 -> [w661]
    tunnel: [w658] -> w84
    tunnel: [w656] -> w83
    tunnel: [w651] -> w82
    tunnel: [w650] -> w69
    tunnel: w80 -> [w648]
    tunnel: w77 -> [w623]
    tunnel: w76 -> [w622]
    tunnel: w74 -> [w615]
    tunnel: [w611] -> w73
    tunnel: [w610] -> w72
    tunnel: [w609] -> w71
    tunnel: [w608] -> w70
    tunnel: w66 -> [w607]
    tunnel: w65 -> [w471]
    tunnel: w32 -> [w606]
    tunnel: [w603] -> w57
    tunnel: [w602] -> _
    tunnel: w63 -> [w598]
    tunnel: [w594] -> w62
    tunnel: w59 -> [w593]
    tunnel: w58 -> [w592]
    tunnel: w32 -> [w473]
    tunnel: [w587] -> w56
    tunnel: [w586] -> w55
    tunnel: w53 -> [w573]
    tunnel: [w569] -> w52
    tunnel: w48 -> [w556]
    tunnel: w47 -> [w555]
    tunnel: [w550] -> w46
    tunnel: [w549] -> w28
    shift-right: [w547] -> w45
    shift-left: w178 -> [w875]
    shift-right: [w546] -> w44
    shift-left: w175 -> [w871]
    tunnel: w32 -> [w539]
    tunnel: [w536] -> w37
    shift-right: [w544] -> w40
    shift-left: w109 -> [w692]
    shift-right: [w543] -> w39
    shift-left: w106 -> [w689]
    tunnel: w38 -> [w538]
    tunnel: w36 -> [w531]
    tunnel: w32 -> [w530]
    tunnel: [w529] -> w35
    tunnel: w33 -> [w522]
    tunnel: w32 -> [w521]
    tunnel: [w520] -> w31
    tunnel: w29 -> [w514]
    tunnel: [w510] -> w27
    tunnel: w25 -> [w509]
    tunnel: [w503] -> w24
    tunnel: w22 -> [w502]
    tunnel: [w497] -> w21
    tunnel: w19 -> [w495]
    tunnel: [w491] -> w18
    tunnel: w16 -> [w487]
    tunnel: [w484] -> w15
    tunnel: w13 -> [w480]
    tunnel: [w477] -> w12
    tunnel: w9 -> [w472]
    tunnel: [w468] -> w8
    tunnel: w4 -> [w467]
    tunnel: w3 -> [w466]
    tunnel: [w462] -> w2
    tunnel: [w458] -> w1
    stop <- w515 stop-if-true
    # "Stop Loop on Error (OR gates)"
    # "Error Stop Loop AND"
    # "Typecast Match AND"
    # "Write Status AND"
    # "READ BOOLS"
    # "READ NUMERICS"
    # "STOP HMI via error or EXIT button"
    # "Check Read status and\nthen convert Variant \nto LabVIEW type (AND gates)"
    # "Sync Read Single"
    n96 = node-c288() -> (w702:errorcluster)  [unwired: 1 in]
    n97 = disable-structure shown="Enabled" {
      frame Enabled {
        n98 = flat-sequence {
          tunnel: [w1193] -> w1137
          tunnel: w1137 -> [w1212]
          frame #0 {
            n99 = disable-structure shown="Enabled" {
              frame Enabled {
                n100 = feedback #1(TRUE) -> (w1139:bool)
                n101 = And(x=TRUE, y=w1139) -> (x .and. y?=w1142:bool)
                n102 = case shown="True" w1142 {
                  tunnel: [FALSE FALSE] -> w1140
                  frame False {
                  }
                  frame True {
                    n103 = local read "Agilent Array"() -> (w1145:T2[])
                    n104 = call "Agilent_Init_Array.vi"("Agilent Array In"=w1145) -> ("Agilent Array Out"=w1146:T2[])
                    n105 = call "Agilent_Arm_Array.vi"("Agilent Array In"=w1146) -> ("Agilent Array Out"=w1144:T2[])
                    n106 = local write "Agilent Array"(w1144) -> ()
                  }
                }
                n107 = feedback-in #1(w1140) -> ()
              }
              frame Disabled {
              }
            }
          }
          frame #1 {
            n108 = case shown="True" "Toggle Scope Scale" {
              frame False {
              }
              frame True {
                n109 = Number To Decimal String(number="CH4 Vertical Units/div") -> (decimal integer string=w1152:string)  [unwired: 1 in]
                n110 = Number To Decimal String(number="Horizontal Units/div") -> (decimal integer string=w1160:string)  [unwired: 1 in]
                n111 = Number To Decimal String(number="CH1 Vertical Units/div") -> (decimal integer string=w1158:string)  [unwired: 1 in]
                n112 = case shown="\"us\"" "Horizontal Units" {
                  tunnel: ["E-06" "E-00" "E-03"] -> w1169
                  frame "us" {
                  }
                  frame "s", Default {
                  }
                  frame "ms" {
                  }
                }
                n113 = Concatenate Strings(":CHAN4:SCAL " ("write buffer"), w1152, "CH4 Vertical Units") -> (w1151:string)
                n114 = Concatenate Strings(":CHAN1:SCAL " ("write buffer"), w1158, "CH1 Vertical Units") -> (w1165:string)
                n115 = Concatenate Strings(":TIM:SCAL " ("write buffer"), w1160, w1169) -> (w1168:string)
                n116 = VISA Open(VISA resource name=refnum<visa-resource-name> "HV_Test_Scope") -> (VISA resource name=w1163:refnum<visa-resource-name>, error out=w1164:errorcluster)  [unwired: 4 in]
                n117 = VISA Write(VISA resource name=w1163, write buffer=w1168, error in (no error)=w1164) -> (VISA resource name out=w1172:refnum<visa-resource-name>, error out=w1171:errorcluster)  [unwired: 1 out]
                n118 = VISA Write(VISA resource name=w1172, write buffer=w1165, error in (no error)=w1171) -> (VISA resource name out=w1157:refnum<visa-resource-name>, error out=w1155:errorcluster)  [unwired: 1 out]
                n119 = VISA Write(VISA resource name=w1157, write buffer=w1151, error in (no error)=w1155) -> (VISA resource name out=w1156:refnum<visa-resource-name>, error out=w1154:errorcluster)  [unwired: 1 out]
                n120 = VISA Close(VISA resource name=w1156, error in (no error)=w1154) -> ()  [unwired: 1 out]
              }
            }
          }
          frame #2 {
            n121 = disable-structure shown="Enabled" {
              frame Enabled {
                n122 = case shown="True" "Stop" {
                  frame False {
                    n123 = disable-structure shown="Disabled" {
                      frame Disabled {
                        n124 = call "Agilent_Init_Array.vi"("Agilent Array In"="Agilent Array") -> ("Agilent Array Out"=w1179:T2[])
                        n125 = local write "Agilent Array"(w1179) -> ()
                      }
                      frame Enabled {
                      }
                    }
                  }
                  frame True {
                    n126 = VISA Open(VISA resource name=refnum<visa-resource-name> "HV_Test_Scope") -> (VISA resource name=w1185:refnum<visa-resource-name>, error out=w1186:errorcluster)  [unwired: 4 in]
                    n127 = VISA Write(VISA resource name=w1185, write buffer=":STOP", error in (no error)=w1186) -> (VISA resource name out=w1183:refnum<visa-resource-name>, error out=w1184:errorcluster)  [unwired: 1 out]
                    n128 = VISA Close(VISA resource name=w1183, error in (no error)=w1184) -> ()  [unwired: 1 out]
                  }
                }
              }
              frame Disabled {
              }
            }
            n129 = case shown="True" "Single" {
              frame False {
              }
              frame True {
                n130 = VISA Open(VISA resource name=refnum<visa-resource-name> "HV_Test_Scope") -> (VISA resource name=w1191:refnum<visa-resource-name>, error out=w1192:errorcluster)  [unwired: 4 in]
                n131 = VISA Write(VISA resource name=w1191, write buffer=":SINGLE", error in (no error)=w1192) -> (VISA resource name out=w1189:refnum<visa-resource-name>, error out=w1190:errorcluster)  [unwired: 1 out]
                n132 = VISA Close(VISA resource name=w1189, error in (no error)=w1190) -> ()  [unwired: 1 out]
              }
            }
          }
          frame #3 {
            n133 = disable-structure shown="Enabled" {
              disable-tunnel: [w1195 w1202 w1207] -> w1193
              frame Disabled {
                n134 = local read "Process Step"() -> (w1194:u8)
                n135 = case shown="1, 6" w1194 {
                  tunnel: [w1196 w1200] -> w1195
                  frame 2..4, Default {
                    n136 = local read "Agilent Array"() -> (w1196:T2[])
                  }
                  frame 1, 6 {
                    n137 = local read "Agilent Array"() -> (w1197:T2[])
                    n138 = local write "Single"(FALSE ("Single")) -> ()
                    n139 = call "Agilent_Arm_Array.vi"("Agilent Array In"=w1197) -> ("Agilent Array Out"=w1200:T2[])
                    n140 = local write "Agilent Array"(w1200) -> ()
                    "Download" <- FALSE ("Downloading")
                  }
                }
              }
              frame Disabled {
                n141 = local read "Process Step"() -> (w1201:u8)
                n142 = case shown="1, 6" w1201 {
                  frame 0, Default {
                  }
                  frame 1, 6 {
                    n143 = local write "Download"(FALSE ("Download")) -> ()
                    n144 = local write "Single"(TRUE ("Single")) -> ()
                  }
                  frame 2 {
                    n145 = local write "Single"(FALSE ("Single")) -> ()
                  }
                }
                n146 = local read "Agilent Array"() -> (w1202:T2[])
              }
              frame Enabled {
                n147 = local read "Process Step"() -> (w1206:u8)
                n148 = case shown="2, 7" w1206 {
                  frame 0, Default {
                  }
                  frame 1, 6 {
                    n149 = local write "Download"(FALSE ("Download")) -> ()
                    n150 = local write "Single"(TRUE ("Single")) -> ()
                  }
                  frame 2, 7 {
                    n151 = local write "Single"(FALSE ("Single")) -> ()
                  }
                }
                n152 = local read "Agilent Array"() -> (w1207:T2[])
              }
            }
          }
          frame #4 {
            n153 = local read "Process Step"() -> (w1211:u8)
            n154 = case shown="0" w1211 {
              tunnel: w1212 -> [_ w1215 w1228]
              frame Default {
              }
              frame 3, 4 {
                n155 = local read "Download"() -> (w1214:bool)
                n156 = Not(x=w1214) -> (.not. x?=w1213:bool)
                n157 = case shown="True" w1213 {
                  tunnel: w1215 -> [_ w1216]
                  frame False {
                  }
                  frame True {
                    n158 = stacked-sequence {
                      tunnel: w1216 -> [_ w1226]
                      frame #0 {
                        n159 = local read "Agilent Array"() -> (w1220:T2[])
                        n160 = Array To Cluster(array=w1220) -> (cluster=w1219:T8)
                        n161 = Unbundle By Name(w1219) -> ("Agilent Array[0].Agilent Control.Desired Samp"=w1217:T9)
                        n162 = call "GF_SetRecordLengthProperly.vi"("Num Samples"=w1217, "VISA resource name"=refnum<visa-resource-name> "HV_Test_Scope") -> ()  [unwired: 1 in, 2 out]
                      }
                      frame #1 {
                        n163 = local write "Download"(TRUE ("Downloading")) -> ()
                        n164 = local write "Single"(FALSE ("Single")) -> ()
                        n165 = call "Agilent_Save_Array.vi"("Agilent Download"=TRUE, "Agilent Array In"=w1226, "File Path"=path "C:/HVTest/Local_Cap_Log_Scope") -> ("Agilent Array Out"=w1224:T2[])  [unwired: 1 in, 1 out]
                        n166 = local write "Agilent Array"(w1224) -> ()
                      }
                    }
                  }
                }
              }
              frame 0 {
                n167 = local read "Maximum Test Number Reached"() -> (w1227:bool)
                n168 = case shown="True" w1227 {
                  tunnel: w1228 -> [_ w1231]
                  frame False {
                  }
                  frame True {
                    n169 = local read "Download"() -> (w1230:bool)
                    n170 = Not(x=w1230) -> (.not. x?=w1229:bool)
                    n171 = case shown="True" w1229 {
                      tunnel: w1231 -> [_ w1232]
                      frame False {
                      }
                      frame True {
                        n172 = stacked-sequence {
                          tunnel: w1232 -> [_ w1242]
                          frame #0 {
                            n173 = local read "Agilent Array"() -> (w1236:T2[])
                            n174 = Array To Cluster(array=w1236) -> (cluster=w1235:T8)
                            n175 = Unbundle By Name(w1235) -> ("Agilent Array[0].Agilent Control.Desired Samp"=w1233:T9)
                            n176 = call "GF_SetRecordLengthProperly.vi"("Num Samples"=w1233, "VISA resource name"=refnum<visa-resource-name> "HV_Test_Scope") -> ()  [unwired: 1 in, 2 out]
                          }
                          frame #1 {
                            n177 = local write "Download"(TRUE ("Downloading")) -> ()
                            n178 = local write "Single"(FALSE ("Single")) -> ()
                            n179 = call "Agilent_Save_Array.vi"("Agilent Download"=TRUE, "Agilent Array In"=w1242, "File Path"=path "C:/HVTest/Local_Cap_Log_Scope") -> ("Agilent Array Out"=w1240:T2[])  [unwired: 1 in, 1 out]
                            n180 = local write "Agilent Array"(w1240) -> ()
                          }
                        }
                      }
                    }
                  }
                }
              }
            }
          }
        }
      }
      frame Disabled {
      }
    }
    n181 = To Word Integer(number="Max Number of Shots (Test intervals)") -> (16bit integer=w525:i16)
    n182 = To Variant(anything=w525) -> (Variant=w524:variant)
    n183 = case shown="1" "HVPS Model" {
      tunnel: ["802L TDK PSU Voltage Rating (abs(Volts))" 12000 50000] -> w816
      tunnel: ["802L TDL PSU Peak Power (J/s)" 9000 9000] -> w839
      frame 2 {
      }
      frame 0, Default {
      }
      frame 1 {
      }
    }
    n184 = call-poly <userlib>:"Write TypeResolved.vi"("Handle"=w471, "SymbolName"=w522, "WData"=w524, "error constant"=w521) -> ("Write Status?"=w517:bool, "Has Matched?"=w518:bool, "error out"=w520:errorcluster)  [unwired: 8 in, 1 out]
    n185 = To Single Precision Float(number="Manual Charge Time (seconds)") -> (single precision float=w533:sgl)
    n186 = To Variant(anything=w533) -> (Variant=w532:variant)
    n187 = And(x="Dump", y="Dump") -> (x .and. y?=w600:bool)
    n188 = To Word Integer(number="Cap 1 Fault Temp (Cel)") -> (16bit integer=w541:i16)
    n189 = To Variant(anything=w600) -> (Variant=w601:variant)
    n190 = flat-sequence {
      tunnel: w872 -> [w1340]
      tunnel: w870 -> [w1341]
      tunnel: w871 -> [w1342]
      tunnel: [w1342] -> w882
      tunnel: [w1341] -> w881
      tunnel: [w1340] -> w880
      tunnel: [w1339] -> w879
      tunnel: w839 -> [w1338]
      tunnel: [w1345] -> w546
      tunnel: [w1348] -> w868
      tunnel: [w1347] -> w869
      tunnel: [w1346] -> w548
      tunnel: w882 -> [w1351]
      tunnel: w881 -> [w1350]
      tunnel: w880 -> [w1349]
      tunnel: w879 -> [w1344]
      tunnel: [w1343] -> w765
      frame #0 {
        # "Write Data"
        n191 = To Long Integer(number=w1338) -> (32bit integer=w1337:i32)
        n192 = To Variant(anything=w1337) -> (Variant=w1339:variant)
      }
      frame #1 {
        # "Resolve To TC"
        n193 = call <userlib>:"Resolve To TC Type.vi"("Handle"=w1349, "TypHdl"=w1350, "WData"=w1344, "error in"=w1351) -> ("Handle"=w1347:u32, "TypHdl"=w1348:u32, "bHasMatched"=w1343:bool, "ADSWData"=w1346:variant, "error out"=w1345:errorcluster)  [unwired: 7 in]
      }
    }
    n194 = flat-sequence {
      tunnel: w951 -> [w1490]
      tunnel: w950 -> [w1491]
      tunnel: w949 -> [w1492]
      tunnel: [w1492] -> w1097
      tunnel: [w1491] -> w1096
      tunnel: [w1490] -> w1095
      tunnel: [w1489] -> w1094
      tunnel: [w1495] -> w712
      tunnel: [w1498] -> w945
      tunnel: [w1497] -> w946
      tunnel: [w1496] -> w886
      tunnel: w1097 -> [w1501]
      tunnel: w1096 -> [w1500]
      tunnel: w1095 -> [w1499]
      tunnel: w1094 -> [w1494]
      tunnel: [w1493] -> w756
      frame #0 {
        # "Write Data"
        n195 = To Single Precision Float(number="Capacitance (uF)") -> (single precision float=w1488:sgl)
        n196 = To Variant(anything=w1488) -> (Variant=w1489:variant)
      }
      frame #1 {
        # "Resolve To TC"
        n197 = call <userlib>:"Resolve To TC Type.vi"("Handle"=w1499, "TypHdl"=w1500, "WData"=w1494, "error in"=w1501) -> ("Handle"=w1497:u32, "TypHdl"=w1498:u32, "bHasMatched"=w1493:bool, "ADSWData"=w1496:variant, "error out"=w1495:errorcluster)  [unwired: 7 in]
      }
    }
    n198 = flat-sequence {
      tunnel: w927 -> [w1460]
      tunnel: w926 -> [w1461]
      tunnel: w925 -> [w1462]
      tunnel: [w1462] -> w1089
      tunnel: [w1461] -> w1088
      tunnel: [w1460] -> w1087
      tunnel: [w1459] -> w1086
      tunnel: w816 -> [w1457]
      tunnel: [w1465] -> w706
      tunnel: [w1468] -> w921
      tunnel: [w1467] -> w922
      tunnel: [w1466] -> w884
      tunnel: w1089 -> [w1471]
      tunnel: w1088 -> [w1470]
      tunnel: w1087 -> [w1469]
      tunnel: w1086 -> [w1464]
      tunnel: [w1463] -> w760
      frame #0 {
        # "Write Data"
        n199 = To Long Integer(number=w1457) -> (32bit integer=w1458:i32)
        n200 = To Variant(anything=w1458) -> (Variant=w1459:variant)
      }
      frame #1 {
        # "Resolve To TC"
        n201 = call <userlib>:"Resolve To TC Type.vi"("Handle"=w1469, "TypHdl"=w1470, "WData"=w1464, "error in"=w1471) -> ("Handle"=w1467:u32, "TypHdl"=w1468:u32, "bHasMatched"=w1463:bool, "ADSWData"=w1466:variant, "error out"=w1465:errorcluster)  [unwired: 7 in]
      }
    }
    n202 = flat-sequence {
      tunnel: w959 -> [w1506]
      tunnel: [w1504] -> _
      tunnel: w957 -> [w1507]
      tunnel: [w1507] -> w1101
      tunnel: [w1504] -> w1100
      tunnel: [w1506] -> w1099
      tunnel: [w1505] -> w1098
      tunnel: w958 -> [w1504]
      tunnel: [w1510] -> w715
      tunnel: [w1513] -> w961
      tunnel: [w1512] -> w960
      tunnel: [w1511] -> w887
      tunnel: w1101 -> [w1516]
      tunnel: w1100 -> [w1515]
      tunnel: w1099 -> [w1514]
      tunnel: w1098 -> [w1509]
      tunnel: [w1508] -> w754
      frame #0 {
        # "Write Data"
        n203 = To Long Integer(number="Cycle Time (Sec)") -> (32bit integer=w1503:i32)
        n204 = To Variant(anything=w1503) -> (Variant=w1505:variant)
      }
      frame #1 {
        # "Resolve To TC"
        n205 = call <userlib>:"Resolve To TC Type.vi"("Handle"=w1514, "TypHdl"=w1515, "WData"=w1509, "error in"=w1516) -> ("Handle"=w1512:u32, "TypHdl"=w1513:u32, "bHasMatched"=w1508:bool, "ADSWData"=w1511:variant, "error out"=w1510:errorcluster)  [unwired: 7 in]
      }
    }
    n206 = flat-sequence {
      tunnel: w939 -> [w1475]
      tunnel: w938 -> [w1476]
      tunnel: w937 -> [w1477]
      tunnel: [w1477] -> w1093
      tunnel: [w1476] -> w1092
      tunnel: [w1475] -> w1091
      tunnel: [w1474] -> w1090
      tunnel: [w1480] -> w709
      tunnel: [w1483] -> w933
      tunnel: [w1482] -> w934
      tunnel: [w1481] -> w885
      tunnel: w1093 -> [w1486]
      tunnel: w1092 -> [w1485]
      tunnel: w1091 -> [w1484]
      tunnel: w1090 -> [w1479]
      tunnel: [w1478] -> w758
      frame #0 {
        # "Write Data"
        n207 = To Long Integer(number="Target Charge Volt (V) - Min 1500V") -> (32bit integer=w1473:i32)
        n208 = To Variant(anything=w1473) -> (Variant=w1474:variant)
      }
      frame #1 {
        # "Resolve To TC"
        n209 = call <userlib>:"Resolve To TC Type.vi"("Handle"=w1484, "TypHdl"=w1485, "WData"=w1479, "error in"=w1486) -> ("Handle"=w1482:u32, "TypHdl"=w1483:u32, "bHasMatched"=w1478:bool, "ADSWData"=w1481:variant, "error out"=w1480:errorcluster)  [unwired: 7 in]
      }
    }
    n210 = flat-sequence {
      tunnel: w915 -> [w1445]
      tunnel: w914 -> [w1446]
      tunnel: w913 -> [w1447]
      tunnel: [w1447] -> w1085
      tunnel: [w1446] -> w1084
      tunnel: [w1445] -> w1083
      tunnel: [w1444] -> w1082
      tunnel: [w1450] -> w703
      tunnel: [w1453] -> w909
      tunnel: [w1452] -> w910
      tunnel: [w1451] -> w883
      tunnel: w1085 -> [w1456]
      tunnel: w1084 -> [w1455]
      tunnel: w1083 -> [w1454]
      tunnel: w1082 -> [w1449]
      tunnel: [w1448] -> w762
      frame #0 {
        # "Write Data"
        n211 = To Single Precision Float(number="Hold Time Before Shot (seconds)") -> (single precision float=w1443:sgl)
        n212 = To Variant(anything=w1443) -> (Variant=w1444:variant)
      }
      frame #1 {
        # "Resolve To TC"
        n213 = call <userlib>:"Resolve To TC Type.vi"("Handle"=w1454, "TypHdl"=w1455, "WData"=w1449, "error in"=w1456) -> ("Handle"=w1452:u32, "TypHdl"=w1453:u32, "bHasMatched"=w1448:bool, "ADSWData"=w1451:variant, "error out"=w1450:errorcluster)  [unwired: 7 in]
      }
    }
    n214 = flat-sequence {
      tunnel: w975 -> [w1355]
      tunnel: w974 -> [w1356]
      tunnel: w973 -> [w1357]
      tunnel: [w1357] -> w1061
      tunnel: [w1356] -> w1060
      tunnel: [w1355] -> w1059
      tunnel: [w1354] -> w1058
      tunnel: [w1360] -> w717
      tunnel: [w1363] -> w969
      tunnel: [w1362] -> w970
      tunnel: [w1361] -> w888
      tunnel: w1061 -> [w1366]
      tunnel: w1060 -> [w1365]
      tunnel: w1059 -> [w1364]
      tunnel: w1058 -> [w1359]
      tunnel: [w1358] -> w753
      frame #0 {
        # "Write Data"
        n215 = And(x="CLEAR FAULT", y="CLEAR FAULT") -> (x .and. y?=w1353:bool)
        n216 = To Variant(anything=w1353) -> (Variant=w1354:variant)
      }
      frame #1 {
        # "Resolve To TC"
        n217 = call <userlib>:"Resolve To TC Type.vi"("Handle"=w1364, "TypHdl"=w1365, "WData"=w1359, "error in"=w1366) -> ("Handle"=w1362:u32, "TypHdl"=w1363:u32, "bHasMatched"=w1358:bool, "ADSWData"=w1361:variant, "error out"=w1360:errorcluster)  [unwired: 7 in]
      }
    }
    n218 = flat-sequence {
      tunnel: w1023 -> [w1415]
      tunnel: w1022 -> [w1416]
      tunnel: w1021 -> [w1417]
      tunnel: [w1417] -> w1077
      tunnel: [w1416] -> w1076
      tunnel: [w1415] -> w1075
      tunnel: [w1414] -> w1074
      tunnel: [w1420] -> w729
      tunnel: [w1423] -> w1017
      tunnel: [w1422] -> w1018
      tunnel: [w1421] -> w892
      tunnel: w1077 -> [w1426]
      tunnel: w1076 -> [w1425]
      tunnel: w1075 -> [w1424]
      tunnel: w1074 -> [w1419]
      tunnel: [w1418] -> w745
      frame #0 {
        # "Write Data"
        n219 = And(x="Hold", y="Hold") -> (x .and. y?=w1413:bool)
        n220 = To Variant(anything=w1413) -> (Variant=w1414:variant)
      }
      frame #1 {
        # "Resolve To TC"
        n221 = call <userlib>:"Resolve To TC Type.vi"("Handle"=w1424, "TypHdl"=w1425, "WData"=w1419, "error in"=w1426) -> ("Handle"=w1422:u32, "TypHdl"=w1423:u32, "bHasMatched"=w1418:bool, "ADSWData"=w1421:variant, "error out"=w1420:errorcluster)  [unwired: 7 in]
      }
    }
    n222 = flat-sequence {
      tunnel: w999 -> [w1385]
      tunnel: w998 -> [w1386]
      tunnel: w997 -> [w1387]
      tunnel: [w1387] -> w1069
      tunnel: [w1386] -> w1068
      tunnel: [w1385] -> w1067
      tunnel: [w1384] -> w1066
      tunnel: [w1390] -> w723
      tunnel: [w1393] -> w993
      tunnel: [w1392] -> w994
      tunnel: [w1391] -> w890
      tunnel: w1069 -> [w1396]
      tunnel: w1068 -> [w1395]
      tunnel: w1067 -> [w1394]
      tunnel: w1066 -> [w1389]
      tunnel: [w1388] -> w749
      frame #0 {
        # "Write Data"
        n223 = And(x="Shot", y="Shot") -> (x .and. y?=w1383:bool)
        n224 = To Variant(anything=w1383) -> (Variant=w1384:variant)
      }
      frame #1 {
        # "Resolve To TC"
        n225 = call <userlib>:"Resolve To TC Type.vi"("Handle"=w1394, "TypHdl"=w1395, "WData"=w1389, "error in"=w1396) -> ("Handle"=w1392:u32, "TypHdl"=w1393:u32, "bHasMatched"=w1388:bool, "ADSWData"=w1391:variant, "error out"=w1390:errorcluster)  [unwired: 7 in]
      }
    }
    n226 = flat-sequence {
      tunnel: w1031 -> [w1431]
      tunnel: [w1427] -> _
      tunnel: w1029 -> [w1432]
      tunnel: [w1432] -> w1081
      tunnel: [w1427] -> w1080
      tunnel: [w1431] -> w1079
      tunnel: [w1430] -> w1078
      tunnel: w1030 -> [w1427]
      tunnel: [w1435] -> w732
      tunnel: [w1438] -> w1033
      tunnel: [w1437] -> w1032
      tunnel: [w1436] -> w893
      tunnel: w1081 -> [w1441]
      tunnel: w1080 -> [w1440]
      tunnel: w1079 -> [w1439]
      tunnel: w1078 -> [w1434]
      tunnel: [w1433] -> w743
      frame #0 {
        # "Write Data"
        n227 = And(x="Manual/Auto", y="Manual/Auto") -> (x .and. y?=w1429:bool)
        n228 = To Variant(anything=w1429) -> (Variant=w1430:variant)
      }
      frame #1 {
        # "Resolve To TC"
        n229 = call <userlib>:"Resolve To TC Type.vi"("Handle"=w1439, "TypHdl"=w1440, "WData"=w1434, "error in"=w1441) -> ("Handle"=w1437:u32, "TypHdl"=w1438:u32, "bHasMatched"=w1433:bool, "ADSWData"=w1436:variant, "error out"=w1435:errorcluster)  [unwired: 7 in]
      }
    }
    n230 = flat-sequence {
      tunnel: w1011 -> [w1400]
      tunnel: w1010 -> [w1401]
      tunnel: w1009 -> [w1402]
      tunnel: [w1402] -> w1073
      tunnel: [w1401] -> w1072
      tunnel: [w1400] -> w1071
      tunnel: [w1399] -> w1070
      tunnel: [w1405] -> w726
      tunnel: [w1408] -> w1005
      tunnel: [w1407] -> w1006
      tunnel: [w1406] -> w891
      tunnel: w1073 -> [w1411]
      tunnel: w1072 -> [w1410]
      tunnel: w1071 -> [w1409]
      tunnel: w1070 -> [w1404]
      tunnel: [w1403] -> w747
      frame #0 {
        # "Write Data"
        n231 = And(x="Charge", y="Charge") -> (x .and. y?=w1398:bool)
        n232 = To Variant(anything=w1398) -> (Variant=w1399:variant)
      }
      frame #1 {
        # "Resolve To TC"
        n233 = call <userlib>:"Resolve To TC Type.vi"("Handle"=w1409, "TypHdl"=w1410, "WData"=w1404, "error in"=w1411) -> ("Handle"=w1407:u32, "TypHdl"=w1408:u32, "bHasMatched"=w1403:bool, "ADSWData"=w1406:variant, "error out"=w1405:errorcluster)  [unwired: 7 in]
      }
    }
    n234 = flat-sequence {
      tunnel: w987 -> [w1370]
      tunnel: w986 -> [w1371]
      tunnel: w985 -> [w1372]
      tunnel: [w1372] -> w1065
      tunnel: [w1371] -> w1064
      tunnel: [w1370] -> w1063
      tunnel: [w1369] -> w1062
      tunnel: [w1375] -> w720
      tunnel: [w1378] -> w981
      tunnel: [w1377] -> w982
      tunnel: [w1376] -> w889
      tunnel: w1065 -> [w1381]
      tunnel: w1064 -> [w1380]
      tunnel: w1063 -> [w1379]
      tunnel: w1062 -> [w1374]
      tunnel: [w1373] -> w751
      frame #0 {
        # "Write Data"
        n235 = And(x="HV Switch Mode", y="HV Switch Mode") -> (x .and. y?=w1368:bool)
        n236 = To Variant(anything=w1368) -> (Variant=w1369:variant)
      }
      frame #1 {
        # "Resolve To TC"
        n237 = call <userlib>:"Resolve To TC Type.vi"("Handle"=w1379, "TypHdl"=w1380, "WData"=w1374, "error in"=w1381) -> ("Handle"=w1377:u32, "TypHdl"=w1378:u32, "bHasMatched"=w1373:bool, "ADSWData"=w1376:variant, "error out"=w1375:errorcluster)  [unwired: 7 in]
      }
    }
    n238 = flat-sequence {
      tunnel: w1047 -> [w1316]
      tunnel: w1046 -> [w1317]
      tunnel: w1045 -> [w1318]
      tunnel: [w1318] -> w807
      tunnel: [w1317] -> w806
      tunnel: [w1316] -> w805
      tunnel: [w1315] -> w804
      tunnel: w807 -> [w1327]
      tunnel: w806 -> [w1326]
      tunnel: w805 -> [w1325]
      tunnel: w804 -> [w1320]
      tunnel: [w1321] -> w735
      tunnel: [w1324] -> w1041
      tunnel: [w1323] -> w1042
      tunnel: [w1322] -> w803
      tunnel: [w1319] -> w741
      frame #0 {
        # "Write Data"
        n239 = And(x="STOP", y="STOP") -> (x .and. y?=w1314:bool)
        n240 = To Variant(anything=w1314) -> (Variant=w1315:variant)
      }
      frame #1 {
        # "Resolve To TC"
        n241 = call <userlib>:"Resolve To TC Type.vi"("Handle"=w1325, "TypHdl"=w1326, "WData"=w1320, "error in"=w1327) -> ("Handle"=w1323:u32, "TypHdl"=w1324:u32, "bHasMatched"=w1319:bool, "ADSWData"=w1322:variant, "error out"=w1321:errorcluster)  [unwired: 7 in]
      }
    }
    n242 = flat-sequence {
      tunnel: w691 -> [w1263]
      tunnel: w690 -> [w1259]
      tunnel: w689 -> [w1264]
      tunnel: [w1264] -> w700
      tunnel: [w1259] -> w699
      tunnel: [w1263] -> w698
      tunnel: [w1262] -> w697
      tunnel: [w1267] -> w543
      tunnel: [w1270] -> w684
      tunnel: [w1269] -> w685
      tunnel: [w1268] -> w688
      tunnel: w700 -> [w1273]
      tunnel: w699 -> [w1272]
      tunnel: w698 -> [w1271]
      tunnel: w697 -> [w1266]
      tunnel: [w1265] -> w682
      frame #0 {
        # "Write Data"
        n243 = And(x="Reset Test Number", y="Reset Test Number") -> (x .and. y?=w1261:bool)
        n244 = To Variant(anything=w1261) -> (Variant=w1262:variant)
      }
      frame #1 {
        # "Resolve To TC"
        n245 = call <userlib>:"Resolve To TC Type.vi"("Handle"=w1271, "TypHdl"=w1272, "WData"=w1266, "error in"=w1273) -> ("Handle"=w1269:u32, "TypHdl"=w1270:u32, "bHasMatched"=w1265:bool, "ADSWData"=w1268:variant, "error out"=w1267:errorcluster)  [unwired: 7 in]
      }
    }
    n246 = flat-sequence {
      tunnel: w1057 -> [w1282]
      tunnel: w1056 -> [w1283]
      tunnel: w1053 -> [w1284]
      tunnel: [w1284] -> w802
      tunnel: [w1283] -> w801
      tunnel: [w1282] -> w800
      tunnel: [w1281] -> w799
      tunnel: [w1279] -> _
      tunnel: [w1279] -> w798
      tunnel: w815 -> [w1279]
      tunnel: w814 -> [w1278]
      tunnel: [w1278] -> w797
      tunnel: w813 -> [w1277]
      tunnel: [w1277] -> w796
      tunnel: w812 -> [w1276]
      tunnel: [w1276] -> w795
      tunnel: w811 -> [w1275]
      tunnel: [w1275] -> w794
      tunnel: ["START"] -> w625
      tunnel: w802 -> [w1298]
      tunnel: w801 -> [w1297]
      tunnel: w800 -> [w1296]
      tunnel: w799 -> [w1291]
      tunnel: [w1292] -> w793
      tunnel: [w1295] -> w792
      tunnel: [w1294] -> w791
      tunnel: [w1293] -> w790
      tunnel: [w1290] -> w789
      tunnel: w798 -> [w1289]
      tunnel: [w1289] -> w788
      tunnel: w797 -> [w1288]
      tunnel: [w1288] -> w787
      tunnel: w796 -> [w1287]
      tunnel: [w1287] -> w786
      tunnel: w795 -> [w1286]
      tunnel: [w1286] -> w785
      tunnel: [w1285] -> w784
      tunnel: w794 -> [w1285]
      tunnel: [w1309] -> w767
      tunnel: [w1310] -> w1055
      tunnel: [w1311] -> w1054
      tunnel: [w1312] -> w738
      tunnel: w793 -> [w1312]
      tunnel: w792 -> [w1311]
      tunnel: w791 -> [w1310]
      tunnel: w790 -> [w1301]
      tunnel: w789 -> [w1309]
      tunnel: w788 -> [w1308]
      tunnel: w787 -> [w1307]
      tunnel: w786 -> [w1306]
      tunnel: w785 -> [w1305]
      tunnel: w784 -> [w1304]
      tunnel: [w1303] -> w810
      tunnel: [w1302] -> w809
      tunnel: [w1300] -> w739
      tunnel: [w1299] -> w782
      frame #0 {
        # "Write Data"
        n247 = And(x="START", y="START") -> (x .and. y?=w1280:bool)
        n248 = To Variant(anything=w1280) -> (Variant=w1281:variant)
      }
      frame #1 {
        # "Resolve To TC"
        n249 = call <userlib>:"Resolve To TC Type.vi"("Handle"=w1296, "TypHdl"=w1297, "WData"=w1291, "error in"=w1298) -> ("Handle"=w1294:u32, "TypHdl"=w1295:u32, "bHasMatched"=w1290:bool, "ADSWData"=w1293:variant, "error out"=w1292:errorcluster)  [unwired: 7 in]
      }
      frame #2 {
        # "Write"
        n250 = call <userlib>:"Send Writer-Request.vi"("Handle"=w1308, "SymbolName"=w1307, "WriterMode"=w1306, "WriteHandle"=w1305, "error constant"=w1304, "ADS Write Data"=w1301) -> ("Handle"=w1303:u32, "WriteHandle"=w1302:u32, "Write status?"=w1299:bool, "error IO"=w1300:errorcluster)  [unwired: 5 in, 1 out]
      }
    }
    n251 = To Variant(anything=w541) -> (Variant=w540:variant)
    n252 = call-poly <userlib>:"Write TypeResolved.vi"("Handle"=w471, "SymbolName"=w531, "WData"=w532, "error constant"=w530) -> ("Write Status?"=w526:bool, "Has Matched?"=w527:bool, "error out"=w529:errorcluster)  [unwired: 8 in, 1 out]
    n253 = call-poly <userlib>:"Write TypeResolved.vi"("Handle"=w471, "SymbolName"=w538, "WData"=w540, "error constant"=w539) -> ("Write Status?"=w535:bool, "Has Matched?"=w537:bool, "error out"=w536:errorcluster)  [unwired: 8 in, 1 out]
    n254 = To Word Integer(number="Soft Dump Temp Thres (Cel)") -> (16bit integer=w489:i16)
    n255 = To Word Integer(number="Load Temp Thres (Cel)") -> (16bit integer=w482:i16)
    n256 = To Unsigned Word Integer(number="Cap Rated Voltage (V)") -> (unsigned 16bit integer=w501:u16)
    n257 = To Variant(anything=w501) -> (Variant=w500:variant)
    n258 = To Word Integer(number="Ambient Temp Thres (Cel)") -> (16bit integer=w475:i16)
    n259 = To Variant(anything=w489) -> (Variant=w488:variant)
    n260 = To Variant(anything=w482) -> (Variant=w481:variant)
    n261 = To Single Precision Float(number="Duty Cycle") -> (single precision float=w584:sgl)
    n262 = And(x="50kV PSU Charger Selected\n(OFF = 12kV Selected, ON = 50kV) Selected", y="50kV PSU Charger Selected\n(OFF = 12kV Selected, ON = 50kV) Selected") -> (x .and. y?=w507:bool)
    n263 = And(x="Voltage Held by PSU", y="Voltage Held by PSU") -> (x .and. y?=w572:bool)
    n264 = And(x="Current Control", y="Current Control") -> (x .and. y?=w591:bool)
    n265 = To Variant(anything=w584) -> (Variant=w588:variant)
    n266 = To Variant(anything=w572) -> (Variant=w570:variant)
    n267 = To Variant(anything=w507) -> (Variant=w508:variant)
    n268 = To Variant(anything=w591) -> (Variant=w589:variant)
    n269 = To Variant(anything=w475) -> (Variant=w474:variant)
    n270 = call-poly <userlib>:"Write TypeResolved.vi"("Handle"=w471, "SymbolName"=w487, "WData"=w488, "error constant"=w473) -> ("Write Status?"=w485:bool, "Has Matched?"=w486:bool, "error out"=w484:errorcluster)  [unwired: 8 in, 1 out]
    n271 = call-poly <userlib>:"Write TypeResolved.vi"("Handle"=w471, "SymbolName"=w480, "WData"=w481, "error constant"=w473) -> ("Write Status?"=w478:bool, "Has Matched?"=w479:bool, "error out"=w477:errorcluster)  [unwired: 8 in, 1 out]
    n272 = call-poly <userlib>:"Write TypeResolved.vi"("Handle"=w471, "SymbolName"=w573, "WData"=w570, "error constant"=w473) -> ("Write Status?"=w563:bool, "Has Matched?"=w564:bool, "error out"=w569:errorcluster)  [unwired: 8 in, 1 out]
    n273 = call-poly <userlib>:"Write TypeResolved.vi"("Handle"=w471, "SymbolName"=w502, "WData"=w500, "error constant"=w473) -> ("Write Status?"=w498:bool, "Has Matched?"=w499:bool, "error out"=w497:errorcluster)  [unwired: 8 in, 1 out]
    n274 = call-poly <userlib>:"Write TypeResolved.vi"("Handle"=w471, "SymbolName"=w509, "WData"=w508, "error constant"=w473) -> ("Write Status?"=w504:bool, "Has Matched?"=w505:bool, "error out"=w503:errorcluster)  [unwired: 8 in, 1 out]
    n275 = call-poly <userlib>:"Write TypeResolved.vi"("Handle"=w471, "SymbolName"=w592, "WData"=w588, "error constant"=w473) -> ("Write Status?"=w562:bool, "Has Matched?"=w565:bool, "error out"=w586:errorcluster)  [unwired: 8 in, 1 out]
    n276 = flat-sequence {
      tunnel: w908 -> [w1664]
      tunnel: w907 -> [w1662]
      tunnel: w906 -> [w1660]
      tunnel: [w1663] -> w1136
      tunnel: [w1661] -> w1135
      tunnel: [w1659] -> w1134
      tunnel: [w1658] -> w1133
      tunnel: [w1657] -> w1132
      tunnel: [w1656] -> w1131
      tunnel: [w1655] -> w1130
      tunnel: [w1654] -> w1129
      tunnel: [w1653] -> w1128
      tunnel: [w1652] -> w1127
      tunnel: [w1651] -> w1126
      tunnel: w904 -> [w1650]
      tunnel: w903 -> [w1649]
      tunnel: w902 -> [w1648]
      tunnel: w901 -> [w1647]
      tunnel: w900 -> [w1646]
      tunnel: w899 -> [w1645]
      tunnel: [w1644] -> w1125
      tunnel: [w1643] -> w1124
      tunnel: [w1642] -> w1123
      tunnel: [w1641] -> w1122
      tunnel: [w1640] -> w1121
      tunnel: [w1639] -> w1120
      tunnel: [w1638] -> w1119
      tunnel: [w1637] -> w1118
      tunnel: [w1636] -> w1117
      tunnel: [w1635] -> w1116
      tunnel: [w1634] -> w1115
      tunnel: [w1633] -> w1114
      tunnel: [w1632] -> w1113
      tunnel: [w1631] -> w1112
      tunnel: [w1630] -> w1111
      tunnel: [w1629] -> w1110
      tunnel: [w1628] -> w1109
      tunnel: [w1627] -> w1108
      tunnel: [w1626] -> w1107
      tunnel: [w1625] -> w1106
      tunnel: [w1624] -> w1105
      tunnel: [w1623] -> w1104
      tunnel: [w1622] -> w1103
      tunnel: [w1621] -> w1102
      tunnel: w866 -> [w1620]
      tunnel: [w1619] -> w865
      tunnel: [w1618] -> w864
      tunnel: [w1617] -> w863
      tunnel: [w1616] -> w862
      tunnel: [w1615] -> w861
      tunnel: w859 -> [w1520]
      tunnel: [w1614] -> w858
      tunnel: w856 -> [w1613]
      tunnel: [w1612] -> w855
      tunnel: [w1611] -> w854
      tunnel: [w1610] -> w853
      tunnel: w852 -> [w1609]
      tunnel: w851 -> [w1608]
      tunnel: [w1607] -> w850
      tunnel: [w1606] -> w849
      tunnel: [w1605] -> w848
      tunnel: [w1604] -> w847
      tunnel: [w1603] -> w846
      tunnel: [w1602] -> w845
      tunnel: [w1601] -> w844
      tunnel: [w1600] -> w843
      tunnel: w835 -> [w1599]
      tunnel: w834 -> [w1598]
      tunnel: w833 -> [w1597]
      tunnel: [w1596] -> w832
      tunnel: [w1595] -> w831
      tunnel: [w1594] -> w830
      tunnel: [w1593] -> w829
      tunnel: [w1592] -> w828
      tunnel: [w1591] -> w827
      tunnel: [w1590] -> w826
      tunnel: [w1589] -> w825
      tunnel: [w1588] -> w824
      tunnel: [w1587] -> w823
      tunnel: [w1586] -> w822
      tunnel: [w1585] -> w821
      tunnel: [w1521] -> _
      tunnel: w808 -> [w1521]
      tunnel: [w1584] -> w676
      tunnel: [w1583] -> w675
      tunnel: [w1582] -> w674
      tunnel: w673 -> [w1581]
      tunnel: [w1580] -> w669
      tunnel: w668 -> [w1579]
      tunnel: [w1578] -> w667
      tunnel: [w1577] -> w666
      tunnel: [w1576] -> w665
      tunnel: [w1575] -> w664
      tunnel: w663 -> [w1574]
      tunnel: w662 -> [w1573]
      tunnel: w661 -> [w1572]
      tunnel: [w1571] -> w660
      tunnel: [w1570] -> w659
      tunnel: [w1569] -> w657
      tunnel: [w1568] -> w655
      tunnel: [w1567] -> w654
      tunnel: [w1566] -> w653
      tunnel: [w1565] -> w652
      tunnel: [w1564] -> w649
      tunnel: w648 -> [w1563]
      tunnel: [w1562] -> w647
      tunnel: [w1561] -> w646
      tunnel: [w1560] -> w645
      tunnel: w623 -> [w1559]
      tunnel: w622 -> [w1558]
      tunnel: [w1557] -> w621
      tunnel: [w1556] -> w620
      tunnel: [w1555] -> w619
      tunnel: [w1554] -> w618
      tunnel: [w1553] -> w617
      tunnel: [w1552] -> w616
      tunnel: w615 -> [w1551]
      tunnel: [w1550] -> w614
      tunnel: [w1549] -> w613
      tunnel: [w1548] -> w612
      tunnel: w598 -> [w1547]
      tunnel: [w1546] -> w597
      tunnel: [w1545] -> w596
      tunnel: [w1544] -> w595
      tunnel: [w1543] -> w558
      tunnel: [w1542] -> w557
      tunnel: w556 -> [w1541]
      tunnel: w555 -> [w1539]
      tunnel: [w1540] -> w554
      tunnel: [w1538] -> w553
      tunnel: [w1537] -> w552
      tunnel: [w1536] -> w551
      tunnel: [w1535] -> w545
      tunnel: w514 -> [w1534]
      tunnel: [w1533] -> w513
      tunnel: [w1532] -> w512
      tunnel: [w1531] -> w511
      tunnel: w495 -> [w1530]
      tunnel: [w1529] -> w494
      tunnel: [w1528] -> w493
      tunnel: [w1527] -> w492
      tunnel: w467 -> [w1526]
      tunnel: w466 -> [w1522]
      tunnel: [w1525] -> w465
      tunnel: [w1523] -> w464
      tunnel: [w1524] -> w463
      tunnel: [w1519] -> w461
      tunnel: [w1518] -> w460
      tunnel: [w1517] -> w459
      tunnel: w1136 -> [w1904]
      tunnel: w1135 -> [w1917]
      tunnel: w1134 -> [_]
      tunnel: w1133 -> [w1903]
      tunnel: w1132 -> [w1902]
      tunnel: w1131 -> [w1733]
      tunnel: [w1832] -> w905
      tunnel: w1130 -> [w1916]
      tunnel: w1129 -> [w1918]
      tunnel: w1128 -> [w1920]
      tunnel: w1127 -> [w1742]
      tunnel: w1126 -> [_]
      tunnel: w1125 -> [w1899]
      tunnel: w1124 -> [w1914]
      tunnel: w1123 -> [w1912]
      tunnel: w1122 -> [w1910]
      tunnel: w1121 -> [w1908]
      tunnel: w1120 -> [w1906]
      tunnel: [w1845] -> w898
      tunnel: w1119 -> [w1898]
      tunnel: w1118 -> [w1897]
      tunnel: w1117 -> [w1896]
      tunnel: w1116 -> [w1895]
      tunnel: w1115 -> [w1894]
      tunnel: w1114 -> [w1893]
      tunnel: w1113 -> [_]
      tunnel: w1112 -> [w1731]
      tunnel: w1111 -> [_]
      tunnel: w1110 -> [w1729]
      tunnel: w1109 -> [_]
      tunnel: w1108 -> [w1727]
      tunnel: w1107 -> [_]
      tunnel: w1106 -> [w1725]
      tunnel: w1105 -> [_]
      tunnel: w1104 -> [w1723]
      tunnel: w1103 -> [_]
      tunnel: w1102 -> [w1721]
      tunnel: [w1847] -> w897
      tunnel: [w1849] -> w896
      tunnel: [w1851] -> w895
      tunnel: [w1853] -> w894
      tunnel: w865 -> [w1719]
      tunnel: w864 -> [w1884]
      tunnel: w863 -> [_]
      tunnel: w862 -> [w1816]
      tunnel: w861 -> [w1880]
      tunnel: [w1836] -> w860
      tunnel: w858 -> [w1883]
      tunnel: [w1834] -> w857
      tunnel: w855 -> [w1882]
      tunnel: w854 -> [w1695]
      tunnel: w853 -> [_]
      tunnel: w850 -> [w1878]
      tunnel: w849 -> [w1877]
      tunnel: w848 -> [w1874]
      tunnel: w847 -> [w1873]
      tunnel: w846 -> [w1872]
      tunnel: w845 -> [w1871]
      tunnel: w844 -> [_]
      tunnel: w843 -> [_]
      tunnel: [w1838] -> w842
      tunnel: [w1840] -> w841
      tunnel: [w1855] -> w838
      tunnel: [w1858] -> w837
      tunnel: [w1857] -> w836
      tunnel: w832 -> [w1869]
      tunnel: w831 -> [w1867]
      tunnel: w830 -> [w1865]
      tunnel: w829 -> [w1737]
      tunnel: w828 -> [w1735]
      tunnel: w827 -> [w1739]
      tunnel: w826 -> [w1864]
      tunnel: w825 -> [w1863]
      tunnel: w824 -> [w1862]
      tunnel: w823 -> [_]
      tunnel: w822 -> [_]
      tunnel: w821 -> [_]
      tunnel: [w1843] -> w820
      tunnel: [w1841] -> w819
      tunnel: [w1830] -> w818
      tunnel: [w1831] -> w516
      tunnel: [w1822] -> w701
      tunnel: [w1824] -> w677
      tunnel: w676 -> [w1741]
      tunnel: w675 -> [w1827]
      tunnel: w674 -> [_]
      tunnel: [w1825] -> w672
      tunnel: w669 -> [w1819]
      tunnel: w667 -> [w1814]
      tunnel: w666 -> [w1811]
      tunnel: w665 -> [w1809]
      tunnel: w664 -> [w1796]
      tunnel: w660 -> [w1717]
      tunnel: w659 -> [w1808]
      tunnel: [w1807] -> w658
      tunnel: w657 -> [w1806]
      tunnel: [w1805] -> w656
      tunnel: w655 -> [w1804]
      tunnel: w654 -> [w1713]
      tunnel: w653 -> [w1803]
      tunnel: w652 -> [w1711]
      tunnel: [w1802] -> w651
      tunnel: [w1801] -> w650
      tunnel: w649 -> [w1715]
      tunnel: [w1800] -> w632
      tunnel: [w1799] -> w630
      tunnel: [w1798] -> w640
      tunnel: w647 -> [w1792]
      tunnel: w646 -> [w1709]
      tunnel: w645 -> [w1794]
      tunnel: [w1793] -> w644
      tunnel: w621 -> [w1788]
      tunnel: w620 -> [w1707]
      tunnel: w619 -> [w1790]
      tunnel: w618 -> [w1789]
      tunnel: w617 -> [w1784]
      tunnel: w616 -> [w1705]
      tunnel: w614 -> [w1770]
      tunnel: w613 -> [w1703]
      tunnel: w612 -> [w1783]
      tunnel: [w1776] -> w611
      tunnel: [w1775] -> w610
      tunnel: [w1774] -> w609
      tunnel: [w1773] -> w608
      tunnel: w597 -> [w1751]
      tunnel: w596 -> [w1768]
      tunnel: w595 -> [w1701]
      tunnel: [w1767] -> w594
      tunnel: w558 -> [w1699]
      tunnel: w557 -> [w1752]
      tunnel: w554 -> [w1747]
      tunnel: w553 -> [w1749]
      tunnel: w552 -> [w1748]
      tunnel: w551 -> [w1697]
      tunnel: [w1744] -> w550
      tunnel: [w1743] -> w549
      tunnel: w545 -> [_]
      tunnel: w513 -> [w1688]
      tunnel: w512 -> [w1692]
      tunnel: w511 -> [w1683]
      tunnel: [w1689] -> w510
      tunnel: w494 -> [w1684]
      tunnel: w493 -> [w1682]
      tunnel: w492 -> [w1681]
      tunnel: [w1680] -> w491
      tunnel: w465 -> [w1677]
      tunnel: w464 -> [w1676]
      tunnel: w463 -> [w1674]
      tunnel: [w1672] -> w462
      tunnel: w461 -> [w1670]
      tunnel: w460 -> [w1669]
      tunnel: w459 -> [w1668]
      tunnel: [w1665] -> w458
      frame #0 {
        # "Read and Resolve Data."
        # "Read/Resolve Symbol N"
        # "Read Data and Resolve Type"
        n277 = call-poly <userlib>:"Read TypeResolved.vi"("Handle"=w1521, "SymbolName"=w1608, "error constant"=w1520) -> ("Handle"=w1601:u32, "Read Status?"=w1606:bool, "RData"=w1602:variant, "error out"=w1605:errorcluster)  [unwired: 9 in]
        n278 = call-poly <userlib>:"Read TypeResolved.vi"("Handle"=w1521, "SymbolName"=w1609, "error constant"=w1520) -> ("Handle"=w1600:u32, "Read Status?"=w1607:bool, "RData"=w1603:variant, "error out"=w1604:errorcluster)  [unwired: 9 in]
        n279 = call-poly <userlib>:"Read TypeResolved.vi"("Handle"=w1521, "SymbolName"=w1662, "error constant"=w1520) -> ("Handle"=w1652:u32, "Read Status?"=w1654:bool, "RData"=w1658:variant, "error out"=w1663:errorcluster)  [unwired: 9 in]
        n280 = call-poly <userlib>:"Read TypeResolved.vi"("Handle"=w1521, "SymbolName"=w1613, "error constant"=w1520) -> ("Handle"=w1610:u32, "Read Status?"=w1612:bool, "RData"=w1611:variant, "error out"=w1615:errorcluster)  [unwired: 9 in]
        n281 = call-poly <userlib>:"Read TypeResolved.vi"("Handle"=w1521, "SymbolName"=w1664, "error constant"=w1520) -> ("Handle"=w1651:u32, "Read Status?"=w1653:bool, "RData"=w1657:variant, "error out"=w1614:errorcluster)  [unwired: 9 in]
        n282 = call-poly <userlib>:"Read TypeResolved.vi"("Handle"=w1521, "SymbolName"=w1522, "error constant"=w1520) -> ("Read Status?"=w1517:bool, "RData"=w1519:variant, "error out"=w1518:errorcluster)  [unwired: 9 in, 1 out]
        n283 = call-poly <userlib>:"Read TypeResolved.vi"("Handle"=w1521, "SymbolName"=w1541, "error constant"=w1520) -> ("Read Status?"=w1540:bool, "RData"=w1543:variant, "error out"=w1542:errorcluster)  [unwired: 9 in, 1 out]
        n284 = call-poly <userlib>:"Read TypeResolved.vi"("Handle"=w1521, "SymbolName"=w1530, "error constant"=w1520) -> ("Read Status?"=w1528:bool, "RData"=w1529:variant, "error out"=w1527:errorcluster)  [unwired: 9 in, 1 out]
        n285 = call-poly <userlib>:"Read TypeResolved.vi"("Handle"=w1521, "SymbolName"=w1526, "error constant"=w1520) -> ("Read Status?"=w1524:bool, "RData"=w1525:variant, "error out"=w1523:errorcluster)  [unwired: 9 in, 1 out]
        n286 = call-poly <userlib>:"Read TypeResolved.vi"("Handle"=w1521, "SymbolName"=w1660, "error constant"=w1520) -> ("Handle"=w1659:u32, "Read Status?"=w1655:bool, "RData"=w1656:variant, "error out"=w1661:errorcluster)  [unwired: 9 in]
        n287 = call-poly <userlib>:"Read TypeResolved.vi"("Handle"=w1521, "SymbolName"=w1534, "error constant"=w1520) -> ("Read Status?"=w1531:bool, "RData"=w1533:variant, "error out"=w1532:errorcluster)  [unwired: 9 in, 1 out]
        n288 = call-poly <userlib>:"Read TypeResolved.vi"("Handle"=w1521, "SymbolName"=w1650, "error constant"=w1520) -> ("Handle"=w1632:u32, "Read Status?"=w1639:bool, "RData"=w1631:variant, "error out"=w1638:errorcluster)  [unwired: 9 in]
        n289 = call-poly <userlib>:"Read TypeResolved.vi"("Handle"=w1521, "SymbolName"=w1551, "error constant"=w1520) -> ("Read Status?"=w1550:bool, "RData"=w1549:variant, "error out"=w1548:errorcluster)  [unwired: 9 in, 1 out]
        n290 = call-poly <userlib>:"Read TypeResolved.vi"("Handle"=w1521, "SymbolName"=w1539, "error constant"=w1520) -> ("Read Status?"=w1537:bool, "RData"=w1536:variant, "error out"=w1538:errorcluster)  [unwired: 9 in, 1 out]
        n291 = call-poly <userlib>:"Read TypeResolved.vi"("Handle"=w1521, "SymbolName"=w1547, "error constant"=w1520) -> ("Read Status?"=w1546:bool, "RData"=w1544:variant, "error out"=w1545:errorcluster)  [unwired: 9 in, 1 out]
        n292 = call-poly <userlib>:"Read TypeResolved.vi"("Handle"=w1521, "SymbolName"=w1648, "error constant"=w1520) -> ("Handle"=w1628:u32, "Read Status?"=w1641:bool, "RData"=w1627:variant, "error out"=w1636:errorcluster)  [unwired: 9 in]
        n293 = call-poly <userlib>:"Read TypeResolved.vi"("Handle"=w1521, "SymbolName"=w1646, "error constant"=w1520) -> ("Handle"=w1624:u32, "Read Status?"=w1643:bool, "RData"=w1623:variant, "error out"=w1634:errorcluster)  [unwired: 9 in]
        n294 = call-poly <userlib>:"Read TypeResolved.vi"("Handle"=w1521, "SymbolName"=w1563, "error constant"=w1520) -> ("Read Status?"=w1562:bool, "RData"=w1561:variant, "error out"=w1560:errorcluster)  [unwired: 9 in, 1 out]
        n295 = call-poly <userlib>:"Read TypeResolved.vi"("Handle"=w1521, "SymbolName"=w1559, "error constant"=w1520) -> ("Read Status?"=w1557:bool, "RData"=w1556:variant, "error out"=w1555:errorcluster)  [unwired: 9 in, 1 out]
        n296 = call-poly <userlib>:"Read TypeResolved.vi"("Handle"=w1521, "SymbolName"=w1558, "error constant"=w1520) -> ("Read Status?"=w1553:bool, "RData"=w1552:variant, "error out"=w1554:errorcluster)  [unwired: 9 in, 1 out]
        n297 = call-poly <userlib>:"Read TypeResolved.vi"("Handle"=w1521, "SymbolName"=w1649, "error constant"=w1520) -> ("Handle"=w1630:u32, "Read Status?"=w1640:bool, "RData"=w1629:variant, "error out"=w1637:errorcluster)  [unwired: 9 in]
        n298 = call-poly <userlib>:"Read TypeResolved.vi"("Handle"=w1521, "SymbolName"=w1647, "error constant"=w1520) -> ("Handle"=w1626:u32, "Read Status?"=w1642:bool, "RData"=w1625:variant, "error out"=w1635:errorcluster)  [unwired: 9 in]
        n299 = call-poly <userlib>:"Read TypeResolved.vi"("Handle"=w1521, "SymbolName"=w1645, "error constant"=w1520) -> ("Handle"=w1622:u32, "Read Status?"=w1644:bool, "RData"=w1621:variant, "error out"=w1633:errorcluster)  [unwired: 9 in]
        n300 = call-poly <userlib>:"Read TypeResolved.vi"("Handle"=w1521, "SymbolName"=w1620, "error constant"=w1520) -> ("Handle"=w1617:u32, "Read Status?"=w1616:bool, "RData"=w1619:variant, "error out"=w1618:errorcluster)  [unwired: 9 in]
        n301 = call-poly <userlib>:"Read TypeResolved.vi"("Handle"=w1521, "SymbolName"=w1579, "error constant"=w1520) -> ("Handle"=w1535:u32, "Read Status?"=w1578:bool, "RData"=w1571:variant, "error out"=w1570:errorcluster)  [unwired: 9 in]
        n302 = call-poly <userlib>:"Read TypeResolved.vi"("Handle"=w1521, "SymbolName"=w1574, "error constant"=w1520) -> ("Read Status?"=w1577:bool, "RData"=w1564:variant, "error out"=w1569:errorcluster)  [unwired: 9 in, 1 out]
        n303 = call-poly <userlib>:"Read TypeResolved.vi"("Handle"=w1521, "SymbolName"=w1572, "error constant"=w1520) -> ("Read Status?"=w1575:bool, "RData"=w1565:variant, "error out"=w1566:errorcluster)  [unwired: 9 in, 1 out]
        n304 = call-poly <userlib>:"Read TypeResolved.vi"("Handle"=w1521, "SymbolName"=w1573, "error constant"=w1520) -> ("Read Status?"=w1576:bool, "RData"=w1567:variant, "error out"=w1568:errorcluster)  [unwired: 9 in, 1 out]
        n305 = call-poly <userlib>:"Read TypeResolved.vi"("Handle"=w1521, "SymbolName"=w1599, "error constant"=w1520) -> ("Handle"=w1587:u32, "Read Status?"=w1596:bool, "RData"=w1592:variant, "error out"=w1588:errorcluster)  [unwired: 9 in]
        n306 = call-poly <userlib>:"Read TypeResolved.vi"("Handle"=w1521, "SymbolName"=w1598, "error constant"=w1520) -> ("Handle"=w1586:u32, "Read Status?"=w1595:bool, "RData"=w1593:variant, "error out"=w1589:errorcluster)  [unwired: 9 in]
        n307 = call-poly <userlib>:"Read TypeResolved.vi"("Handle"=w1521, "SymbolName"=w1581, "error constant"=w1520) -> ("Handle"=w1582:u32, "Read Status?"=w1580:bool, "RData"=w1584:variant, "error out"=w1583:errorcluster)  [unwired: 9 in]
        n308 = call-poly <userlib>:"Read TypeResolved.vi"("Handle"=w1521, "SymbolName"=w1597, "error constant"=w1520) -> ("Handle"=w1585:u32, "Read Status?"=w1594:bool, "RData"=w1591:variant, "error out"=w1590:errorcluster)  [unwired: 9 in]
      }
      frame #1 {
        # "Cast Symbol N to LabVIEW Type"
        # "Variant To Data"
        n309 = To Variant(anything=w1684) -> (Variant=w1685:variant)
        n310 = To Variant(anything=w1677) -> (Variant=w1679:variant)
        n311 = To Variant(anything=w1670) -> (Variant=w1678:variant)
        n312 = To Variant(anything=w1697) -> (Variant=w1696:variant)
        n313 = To Variant(anything=w1739) -> (Variant=w1738:variant)
        n314 = To Variant(anything=w1711) -> (Variant=w1710:variant)
        n315 = To Variant(anything=w1737) -> (Variant=w1736:variant)
        n316 = To Variant(anything=w1705) -> (Variant=w1704:variant)
        n317 = To Variant(anything=w1707) -> (Variant=w1706:variant)
        n318 = To Variant(anything=w1699) -> (Variant=w1698:variant)
        n319 = To Variant(anything=w1709) -> (Variant=w1708:variant)
        n320 = To Variant(anything=w1701) -> (Variant=w1700:variant)
        n321 = To Variant(anything=w1703) -> (Variant=w1702:variant)
        n322 = To Variant(anything=w1735) -> (Variant=w1734:variant)
        n323 = To Variant(anything=w1719) -> (Variant=w1718:variant)
        n324 = To Variant(anything=w1717) -> (Variant=w1716:variant)
        n325 = To Variant(anything=w1715) -> (Variant=w1714:variant)
        n326 = To Variant(anything=w1729) -> (Variant=w1728:variant)
        n327 = To Variant(anything=w1695) -> (Variant=w1694:variant)
        n328 = To Variant(anything=w1713) -> (Variant=w1712:variant)
        n329 = To Variant(anything=w1733) -> (Variant=w1732:variant)
        n330 = To Variant(anything=w1731) -> (Variant=w1730:variant)
        n331 = To Variant(anything=w1721) -> (Variant=w1720:variant)
        n332 = To Variant(anything=w1741) -> (Variant=w1740:variant)
        n333 = To Variant(anything=w1727) -> (Variant=w1726:variant)
        n334 = To Variant(anything=w1723) -> (Variant=w1722:variant)
        n335 = And(x=w1683, y=w1682) -> (x .and. y?=w1673:bool)
        n336 = To Variant(anything=w1725) -> (Variant=w1724:variant)
        n337 = Variant To Data(error in=w1692, Variant=w1688) -> (data=→"Spark Gap Voltage":i16, error out=w1689:errorcluster)  [unwired: 1 in]
        n338 = And(x=w1747, y=w1748) -> (x .and. y?=w1691:bool)
        n339 = Variant To Data(error in=w1681, Variant=w1685) -> (data=→"Target Voltage Exceeded\nCap Rating Voltage":bool, error out=w1680:errorcluster)  [unwired: 1 in]
        n340 = Variant To Data(error in=w1676, Variant=w1679) -> (data=→"All Temp In Range":bool, error out=w1672:errorcluster)  [unwired: 1 in]
        n341 = Variant To Data(error in=w1669, Variant=w1678) -> (data=→"Load Temp Fault":bool, error out=w1665:errorcluster)  [unwired: 1 in]
        n342 = Variant To Data(error in=w1752, Variant=w1698) -> (data=→"Test Interval (Sec)":i32, error out=w1744:errorcluster)  [unwired: 1 in]
        n343 = Variant To Data(error in=w1749, Variant=w1696) -> (data=→"Test Interval Fault":bool, error out=w1743:errorcluster)  [unwired: 1 in]
        n344 = And(x=w1673, y=w1674) -> (x .and. y?=w1667:bool)
        n345 = And(x=w1667, y=w1668) -> (x .and. y?=w1666:bool)
        n346 = Variant To Data(error in=w1827, Variant=w1740) -> (data=→"Cap 1 Voltage (HVPS)":i16, error out=w1825:errorcluster)  [unwired: 1 in]
        n347 = Variant To Data(error in=w1898, Variant=w1730) -> (data=→"Discharge Fault":bool, error out=w1847:errorcluster)  [unwired: 1 in]
        n348 = Variant To Data(error in=w1917, Variant=w1732) -> (data=→"Charge Fault":bool, error out=w1845:errorcluster)  [unwired: 1 in]
        n349 = Variant To Data(error in=w1896, Variant=w1726) -> (data=→"Cap 1 Temp\nExceeded Fault":bool, error out=w1851:errorcluster)  [unwired: 1 in]
        n350 = Variant To Data(error in=w1897, Variant=w1728) -> (data=→"Hold Fault":bool, error out=w1849:errorcluster)  [unwired: 1 in]
        n351 = Variant To Data(error in=w1864, Variant=w1738) -> (data=→"Load Temperature":i16, error out=w1830:errorcluster)  [unwired: 1 in]
        n352 = Variant To Data(error in=w1895, Variant=w1724) -> (data=→"Ambient Temp\nExceeded Fault":bool, error out=w1853:errorcluster)  [unwired: 1 in]
        n353 = Variant To Data(error in=w1894, Variant=w1722) -> (data=→"PSU Fault":bool, error out=w1855:errorcluster)  [unwired: 1 in]
        n354 = Variant To Data(error in=w1893, Variant=w1720) -> (data=→"Control Sys Fault":bool, error out=w1857:errorcluster)  [unwired: 1 in]
        n355 = Variant To Data(error in=w1884, Variant=w1718) -> (data=→"test Running":bool, error out=w1858:errorcluster)  [unwired: 1 in]
        n356 = Variant To Data(error in=w1862, Variant=w1734) -> (data=→"Ambient Temp":i16, error out=w1843:errorcluster)  [unwired: 1 in]
        n357 = Variant To Data(error in=w1803, Variant=w1710) -> (data=w1798:bool, error out=w1801:errorcluster)  [unwired: 1 in]
        "Soft Exception" <- w1798
        n358 = Variant To Data(error in=w1794, Variant=w1708) -> (data=w1693:bool, error out=w1776:errorcluster)  [unwired: 1 in]
        "EOC" <- w1693
        n359 = Variant To Data(error in=w1873, Variant=w1872) -> (data=w1782:i16, error out=w1838:errorcluster)  [unwired: 1 in]
        "Cap 1 Voltage" <- w1782
        n360 = Variant To Data(error in=w1863, Variant=w1736) -> (data=→"Soft Dump Temp":i16, error out=w1841:errorcluster)  [unwired: 1 in]
        n361 = Variant To Data(error in=w1808, Variant=w1716) -> (data=w1793:bool, error out=w1807:errorcluster)  [unwired: 1 in]
        "Softdump FB Fault" <- w1793
        n362 = Variant To Data(error in=w1804, Variant=w1712) -> (data=w1799:bool, error out=w1802:errorcluster)  [unwired: 1 in]
        "PSU HV FB Fault" <- w1799
        n363 = Variant To Data(error in=w1790, Variant=w1706) -> (data=w1764:bool, error out=w1775:errorcluster)  [unwired: 1 in]
        "SCR Ready" <- w1764
        n364 = Variant To Data(error in=w1789, Variant=w1704) -> (data=→"Maximum Test Number Reached":bool, error out=w1774:errorcluster)  [unwired: 1 in]
        n365 = Variant To Data(error in=w1806, Variant=w1714) -> (data=w1800:bool, error out=w1805:errorcluster)  [unwired: 1 in]
        "Charge FB Fault" <- w1800
        n366 = Variant To Data(error in=w1768, Variant=w1700) -> (data=w1765:bool, error out=w1767:errorcluster)  [unwired: 1 in]
        "Scope Trig" <- w1765
        n367 = Variant To Data(error in=w1880, Variant=w1694) -> (data=w1766:u8, error out=w1836:errorcluster)  [unwired: 1 in]
        "Process Step" <- w1766
        n368 = And(x=w1691, y=w1666) -> (x .and. y?=w1690:bool)
        n369 = And(x=w1751, y=w1690) -> (x .and. y?=w1750:bool)
        n370 = And(x=w1770, y=w1750) -> (x .and. y?=w1769:bool)
        n371 = And(x=w1784, y=w1769) -> (x .and. y?=w1785:bool)
        n372 = And(x=w1788, y=w1785) -> (x .and. y?=w1787:bool)
        n373 = And(x=w1792, y=w1787) -> (x .and. y?=w1791:bool)
        n374 = And(x=w1796, y=w1791) -> (x .and. y?=w1795:bool)
        n375 = And(x=w1809, y=w1795) -> (x .and. y?=w1810:bool)
        n376 = And(x=w1811, y=w1810) -> (x .and. y?=w1812:bool)
        n377 = And(x=w1814, y=w1812) -> (x .and. y?=w1813:bool)
        n378 = And(x=w1816, y=w1813) -> (x .and. y?=w1815:bool)
        n379 = And(x=w1899, y=w1815) -> (x .and. y?=w1915:bool)
        n380 = And(x=w1914, y=w1915) -> (x .and. y?=w1913:bool)
        n381 = And(x=w1912, y=w1913) -> (x .and. y?=w1911:bool)
        n382 = And(x=w1910, y=w1911) -> (x .and. y?=w1909:bool)
        n383 = And(x=w1908, y=w1909) -> (x .and. y?=w1907:bool)
        n384 = And(x=w1906, y=w1907) -> (x .and. y?=w1905:bool)
        n385 = And(x=w1916, y=w1905) -> (x .and. y?=w1870:bool)
        n386 = And(x=w1869, y=w1870) -> (x .and. y?=w1868:bool)
        n387 = And(x=w1867, y=w1868) -> (x .and. y?=w1866:bool)
        n388 = And(x=w1865, y=w1866) -> (x .and. y?=w1818:bool)
        n389 = And(x=w1819, y=w1818) -> (x .and. y?=w1817:bool)
        n390 = And(x=w1877, y=w1817) -> (x .and. y?=w1876:bool)
        n391 = And(x=w1878, y=w1876) -> (x .and. y?=w1875:bool)
        n392 = And(x=w1882, y=w1875) -> (x .and. y?=w1881:bool)
        n393 = And(x=w1920, y=w1881) -> (x .and. y?=w1919:bool)
        n394 = And(x=w1918, y=w1919) -> (x .and. y?=→"Read Status":bool)
        n395 = Variant To Data(error in=w1874, Variant=w1871) -> (data=→"Cap 1 Temperature":i16, error out=w1840:errorcluster)  [unwired: 1 in]
        n396 = Variant To Data(error in=w1783, Variant=w1702) -> (data=w1772:i16, error out=w1773:errorcluster)  [unwired: 1 in]
        "Expected Voltage" <- w1772
        n397 = Variant To Data(error in=w1904, Variant=w1903) -> (data=→"Estimated Charge Time (seconds)":sgl, error out=w1832:errorcluster)  [unwired: 1 in]
        n398 = To Double Precision Float(number=w1782) -> (double precision float=→"Waveform Chart - Capacitor Voltage (Probe, abs(Volts))":dbl)
        n399 = Variant To Data(error in=w1883, Variant=w1902) -> (data=→"Shot Number":i16, error out=w1834:errorcluster)  [unwired: 1 in]
        n400 = case shown="True" "Log Temperature Data" {
          tunnel: [errorcluster {"status"=FALSE, "code"=0, "source"=""} ("error out") w1931] -> w1824
          frame False {
          }
          frame True {
            n401 = local read "Cap 1 Temperature"() -> (w1932:i16)
            n402 = local read "test Running"() -> (w1930:bool)
            n403 = call "Write To Measurement File2"("Signals"=w1932, "Enable"=w1930, "Filename"="Capacitor Temperature Data Log File Path (.xlsx)") -> ("error out"=w1931:errorcluster)  [unwired: 14 in, 2 out]
          }
        }
        n404 = case shown="2" w1766 {
          tunnel: ["Charge" "Current Controlled Charge" "Hold - Ready for Shot" "Hold - Cap Open Circuited" "Shot" "Wait" "Dump" "Error" "Wait"] -> w1879
          tunnel: [TRUE TRUE TRUE TRUE TRUE TRUE FALSE FALSE FALSE] -> w1762
          tunnel: [FALSE ("Reset") FALSE ("Reset") FALSE ("Reset") FALSE ("Reset") TRUE ("Reset") FALSE ("Reset") FALSE ("Reset") TRUE ("Reset") FALSE ("Reset")] -> _
          frame 1 {
          }
          frame 6 {
          }
          frame 2 {
          }
          frame 7 {
          }
          frame 3 {
          }
          frame 4 {
          }
          frame 5 {
          }
          frame 99 {
          }
          frame 0, Default {
          }
        }
        "Test State" <- w1879
        n405 = local write "Scope Trig"(w1765) -> ()
        n406 = local read "Cap 1 Voltage"() -> (w1754:i16)
        n407 = case shown="True" "Log Capacitor Voltage" {
          tunnel: [errorcluster {"status"=FALSE, "code"=0, "source"=""} ("error out") w1928] -> w1822
          tunnel: w1782 -> [_ w1927]
          tunnel: w1762 -> [_ w1926]
          frame False {
          }
          frame True {
            n408 = local read "test Running"() -> (w1923:bool)
            n409 = And(x=w1926, y=w1923) -> (x .and. y?=w1924:bool)
            n410 = call "Write To Measurement File"("Signals"=w1927, "Enable"=w1924, "Filename"="Capacitor Voltage Data Log File Path (.xlsx)") -> ("error out"=w1928:errorcluster)  [unwired: 14 in, 2 out]
          }
        }
        n411 = Not(x=w1693) -> (.not. x?=w1780:bool)
        n412 = To Double Precision Float(number=w1754) -> (double precision float=w1778:dbl)
        n413 = To Double Precision Float(number=w1772) -> (double precision float=w1771:dbl)
        n414 = Boolean To (0,1)(Boolean=w1780) -> (0, 1=→"EOC":i16)
        n415 = Or(x=w1857, y=w1858) -> (x .or. y?=w1856:bool)
        n416 = Or(x=w1855, y=w1856) -> (x .or. y?=w1854:bool)
        n417 = Or(x=w1853, y=w1854) -> (x .or. y?=w1852:bool)
        n418 = Or(x=w1851, y=w1852) -> (x .or. y?=w1850:bool)
        n419 = Or(x=w1849, y=w1850) -> (x .or. y?=w1848:bool)
        n420 = Or(x=w1847, y=w1848) -> (x .or. y?=w1846:bool)
        n421 = Or(x=w1845, y=w1846) -> (x .or. y?=w1844:bool)
        n422 = Or(x=w1843, y=w1844) -> (x .or. y?=w1842:bool)
        n423 = Or(x=w1841, y=w1842) -> (x .or. y?=w1829:bool)
        n424 = Or(x=w1830, y=w1829) -> (x .or. y?=w1823:bool)
        n425 = Boolean To (0,1)(Boolean=w1764) -> (0, 1=→"SCR FB":i16)
        n426 = Bundle(w1778, w1771) -> (→"Capacitor Voltage":cluster{dbl, dbl})  [unwired: 1 in]
        n427 = local write "Process Step"(w1766) -> ()
        n428 = local read "Scope Trig"() -> (w1757:bool)
        n429 = local read "Test Interval (Sec)"() -> (w1760:i32)
        n430 = Not(x=w1757) -> (.not. x?=w1756:bool)
        n431 = call "Elapsed Time"("Time Target (s)"=w1760, "Reset"=w1756) -> ("Elapsed Time Text"=w1759:string)  [unwired: 10 in, 7 out]
        n432 = String Subset(string=w1759, offset (0)=2) -> (substring=→"Time Since Last Shot":string)  [unwired: 1 in]
        n433 = Or(x=w1824, y=w1823) -> (x .or. y?=w1821:bool)
        n434 = Or(x=w1822, y=w1821) -> (x .or. y?=w1820:bool)
        n435 = Or(x=w1840, y=w1820) -> (x .or. y?=w1839:bool)
        n436 = Or(x=w1838, y=w1839) -> (x .or. y?=w1837:bool)
        n437 = Or(x=w1836, y=w1837) -> (x .or. y?=w1835:bool)
        n438 = Or(x=w1834, y=w1835) -> (x .or. y?=w1833:bool)
        n439 = Or(x=w1832, y=w1833) -> (x .or. y?=w1831:bool)
        n440 = case shown="True" w1693 {
          frame False {
          }
          frame True {
            n441 = local write "Single"(TRUE) -> ()
          }
        }
        "Internal TwinCAT Handle ID Maps" <- w1742
      }
    }
    n442 = call-poly <userlib>:"Write TypeResolved.vi"("Handle"=w471, "SymbolName"=w472, "WData"=w474, "error constant"=w473) -> ("Write Status?"=w469:bool, "Has Matched?"=w470:bool, "error out"=w468:errorcluster)  [unwired: 8 in, 1 out]
    n443 = call-poly <userlib>:"Write TypeResolved.vi"("Handle"=w471, "SymbolName"=w593, "WData"=w589, "error constant"=w473) -> ("Write Status?"=w561:bool, "Has Matched?"=w566:bool, "error out"=w587:errorcluster)  [unwired: 8 in, 1 out]
    n444 = call-poly <userlib>:"Write TypeResolved.vi"("Handle"=w471, "SymbolName"=w607, "WData"=w601, "error constant"=w606) -> ("Handle"=w602:u32, "Write Status?"=w560:bool, "Has Matched?"=w568:bool, "error out"=w603:errorcluster)  [unwired: 8 in]
    n445 = call <userlib>:"Send Writer-Request.vi"("Handle"=w1052, "SymbolName"=w1051, "WriterMode"=w1050, "WriteHandle"=w1049, "error constant"=w1048, "ADS Write Data"=w803) -> ("Handle"=w1044:u32, "WriteHandle"=w1043:u32, "Write status?"=w781:bool, "error IO"=w736:errorcluster)  [unwired: 5 in, 1 out]
    n446 = call <userlib>:"Send Writer-Request.vi"("Handle"=w968, "SymbolName"=w967, "WriterMode"=w966, "WriteHandle"=w964, "error constant"=w965, "ADS Write Data"=w887) -> ("Handle"=w963:u32, "WriteHandle"=w962:u32, "Write status?"=w583:bool, "error IO"=w716:errorcluster)  [unwired: 5 in, 1 out]
    n447 = call <userlib>:"Send Writer-Request.vi"("Handle"=w878, "SymbolName"=w877, "WriterMode"=w876, "WriteHandle"=w867, "error constant"=w875, "ADS Write Data"=w548) -> ("Handle"=w874:u32, "WriteHandle"=w873:u32, "Write status?"=w578:bool, "error IO"=w547:errorcluster)  [unwired: 5 in, 1 out]
    n448 = call <userlib>:"Send Writer-Request.vi"("Handle"=w956, "SymbolName"=w955, "WriterMode"=w954, "WriteHandle"=w953, "error constant"=w952, "ADS Write Data"=w886) -> ("Handle"=w948:u32, "WriteHandle"=w947:u32, "Write status?"=w582:bool, "error IO"=w713:errorcluster)  [unwired: 5 in, 1 out]
    n449 = call <userlib>:"Send Writer-Request.vi"("Handle"=w932, "SymbolName"=w931, "WriterMode"=w930, "WriteHandle"=w929, "error constant"=w928, "ADS Write Data"=w884) -> ("Handle"=w924:u32, "WriteHandle"=w923:u32, "Write status?"=w580:bool, "error IO"=w707:errorcluster)  [unwired: 5 in, 1 out]
    n450 = call <userlib>:"Send Writer-Request.vi"("Handle"=w944, "SymbolName"=w943, "WriterMode"=w942, "WriteHandle"=w941, "error constant"=w940, "ADS Write Data"=w885) -> ("Handle"=w936:u32, "WriteHandle"=w935:u32, "Write status?"=w581:bool, "error IO"=w710:errorcluster)  [unwired: 5 in, 1 out]
    n451 = call <userlib>:"Send Writer-Request.vi"("Handle"=w920, "SymbolName"=w919, "WriterMode"=w918, "WriteHandle"=w917, "error constant"=w916, "ADS Write Data"=w883) -> ("Handle"=w912:u32, "WriteHandle"=w911:u32, "Write status?"=w579:bool, "error IO"=w704:errorcluster)  [unwired: 5 in, 1 out]
    n452 = call <userlib>:"Send Writer-Request.vi"("Handle"=w1040, "SymbolName"=w1039, "WriterMode"=w1038, "WriteHandle"=w1036, "error constant"=w1037, "ADS Write Data"=w893) -> ("Handle"=w1035:u32, "WriteHandle"=w1034:u32, "Write status?"=w769:bool, "error IO"=w733:errorcluster)  [unwired: 5 in, 1 out]
    n453 = call <userlib>:"Send Writer-Request.vi"("Handle"=w980, "SymbolName"=w979, "WriterMode"=w978, "WriteHandle"=w977, "error constant"=w976, "ADS Write Data"=w888) -> ("Handle"=w972:u32, "WriteHandle"=w971:u32, "Write status?"=w779:bool, "error IO"=w718:errorcluster)  [unwired: 5 in, 1 out]
    n454 = call <userlib>:"Send Writer-Request.vi"("Handle"=w1028, "SymbolName"=w1027, "WriterMode"=w1026, "WriteHandle"=w1025, "error constant"=w1024, "ADS Write Data"=w892) -> ("Handle"=w1020:u32, "WriteHandle"=w1019:u32, "Write status?"=w771:bool, "error IO"=w730:errorcluster)  [unwired: 5 in, 1 out]
    n455 = call <userlib>:"Send Writer-Request.vi"("Handle"=w1004, "SymbolName"=w1003, "WriterMode"=w1002, "WriteHandle"=w1001, "error constant"=w1000, "ADS Write Data"=w890) -> ("Handle"=w996:u32, "WriteHandle"=w995:u32, "Write status?"=w775:bool, "error IO"=w724:errorcluster)  [unwired: 5 in, 1 out]
    n456 = call <userlib>:"Send Writer-Request.vi"("Handle"=w1016, "SymbolName"=w1015, "WriterMode"=w1014, "WriteHandle"=w1013, "error constant"=w1012, "ADS Write Data"=w891) -> ("Handle"=w1008:u32, "WriteHandle"=w1007:u32, "Write status?"=w773:bool, "error IO"=w727:errorcluster)  [unwired: 5 in, 1 out]
    n457 = call <userlib>:"Send Writer-Request.vi"("Handle"=w992, "SymbolName"=w991, "WriterMode"=w990, "WriteHandle"=w989, "error constant"=w988, "ADS Write Data"=w889) -> ("Handle"=w984:u32, "WriteHandle"=w983:u32, "Write status?"=w777:bool, "error IO"=w721:errorcluster)  [unwired: 5 in, 1 out]
    n458 = call <userlib>:"Send Writer-Request.vi"("Handle"=w696, "SymbolName"=w695, "WriterMode"=w694, "WriteHandle"=w693, "error constant"=w692, "ADS Write Data"=w688) -> ("Handle"=w687:u32, "WriteHandle"=w686:u32, "Write status?"=w680:bool, "error IO"=w544:errorcluster)  [unwired: 5 in, 1 out]
    n459 = Compound Arithmetic op=AND(w568, w566, w565, w564, w505, w499, w486, w479, w470) -> (w567:bool)
    n460 = And(x=w537, y=w567) -> (x .and. y?=w604:bool)
    n461 = And(x=w527, y=w604) -> (x .and. y?=w678:bool)
    n462 = And(x=w765, y=w678) -> (x .and. y?=w764:bool)
    n463 = And(x=w518, y=w764) -> (x .and. y?=w763:bool)
    n464 = And(x=w762, y=w763) -> (x .and. y?=w761:bool)
    n465 = And(x=w760, y=w761) -> (x .and. y?=w759:bool)
    n466 = And(x=w758, y=w759) -> (x .and. y?=w757:bool)
    n467 = And(x=w756, y=w757) -> (x .and. y?=w755:bool)
    n468 = And(x=w754, y=w755) -> (x .and. y?=w671:bool)
    n469 = And(x=w682, y=w671) -> (x .and. y?=w683:bool)
    n470 = And(x=w753, y=w683) -> (x .and. y?=w752:bool)
    n471 = And(x=w751, y=w752) -> (x .and. y?=w750:bool)
    n472 = And(x=w749, y=w750) -> (x .and. y?=w748:bool)
    n473 = And(x=w747, y=w748) -> (x .and. y?=w746:bool)
    n474 = And(x=w745, y=w746) -> (x .and. y?=w744:bool)
    n475 = And(x=w743, y=w744) -> (x .and. y?=w742:bool)
    n476 = And(x=w741, y=w742) -> (x .and. y?=w740:bool)
    n477 = And(x=w767, y=w740) -> (x .and. y?=→"bHasMached":bool)
    n478 = Compound Arithmetic op=AND(w560, w561, w562, w563, w504, w498, w485, w478, w469) -> (w559:bool)
    n479 = And(x=w535, y=w559) -> (x .and. y?=w605:bool)
    n480 = And(x=w526, y=w605) -> (x .and. y?=w575:bool)
    n481 = Compound Arithmetic op=AND(w583, w582, w581, w580, w579, w517, w578) -> (w577:bool)
    n482 = Not(x=w577) -> (.not. x?=w576:bool)
    n483 = And(x=w576, y=w575) -> (x .and. y?=w574:bool)
    n484 = And(x=w680, y=w574) -> (x .and. y?=w681:bool)
    n485 = And(x=w779, y=w681) -> (x .and. y?=w778:bool)
    n486 = And(x=w777, y=w778) -> (x .and. y?=w776:bool)
    n487 = And(x=w775, y=w776) -> (x .and. y?=w774:bool)
    n488 = And(x=w773, y=w774) -> (x .and. y?=w772:bool)
    n489 = And(x=w771, y=w772) -> (x .and. y?=w770:bool)
    n490 = And(x=w769, y=w770) -> (x .and. y?=w768:bool)
    n491 = And(x=w781, y=w768) -> (x .and. y?=w780:bool)
    n492 = And(x=w782, y=w780) -> (x .and. y?=→"Write Status":bool)
    n493 = feedback #2(TRUE) -> (w627:bool)
    n494 = And(x=w627, y=w630) -> (x .and. y?=w629:bool)
    n495 = feedback #3(TRUE) -> (w637:bool)
    n496 = And(x=w637, y=w640) -> (x .and. y?=w639:bool)
    n497 = feedback #4(TRUE) -> (w641:bool)
    n498 = And(x=w641, y=w644) -> (x .and. y?=w643:bool)
    n499 = feedback #5(TRUE) -> (w633:bool)
    n500 = And(x=w633, y=w632) -> (x .and. y?=w634:bool)
    n501 = case shown="True" w634 {
      tunnel: [w1247 FALSE] -> w624
      tunnel: w625 -> [w1249 _]
      frame False {
        n502 = Or(x=w1249, y=FALSE) -> (x .or. y?=w1247:bool)
      }
      frame True {
        n503 = call "Charge relay error"() -> ()  [unwired: 10 in, 2 out]
      }
    }
    n504 = feedback-in #5(w624) -> ()
    n505 = case shown="True" w629 {
      tunnel: [w1245 FALSE] -> w628
      tunnel: w624 -> [w1243 _]
      frame False {
        n506 = Or(x=w1243, y=FALSE) -> (x .or. y?=w1245:bool)
      }
      frame True {
        n507 = call "PSU HV error"() -> ()  [unwired: 10 in, 2 out]
      }
    }
    n508 = feedback-in #2(w628) -> ()
    n509 = case shown="True" w643 {
      tunnel: [w1256 FALSE] -> w642
      tunnel: w625 -> [w1255 _]
      frame False {
        n510 = Or(x=w1255, y=FALSE) -> (x .or. y?=w1256:bool)
      }
      frame True {
        n511 = call "Softdump error"() -> ()  [unwired: 10 in, 2 out]
      }
    }
    n512 = feedback-in #4(w642) -> ()
    n513 = case shown="True" w639 {
      tunnel: [w1251 FALSE] -> w638
      tunnel: w624 -> [w1252 _]
      frame False {
        n514 = Or(x=w1252, y=FALSE) -> (x .or. y?=w1251:bool)
      }
      frame True {
        n515 = call "Soft Exception"() -> ()  [unwired: 10 in, 2 out]
      }
    }
    n516 = feedback-in #3(w638) -> ()
    n517 = Compound Arithmetic op=OR(w702, w739, w738) -> (w737:bool)
    n518 = Compound Arithmetic op=OR(w737, w736, w735) -> (w734:bool)
    n519 = Compound Arithmetic op=OR(w734, w733, w732) -> (w731:bool)
    n520 = Compound Arithmetic op=OR(w731, w730, w729) -> (w728:bool)
    n521 = Compound Arithmetic op=OR(w728, w727, w726) -> (w725:bool)
    n522 = Compound Arithmetic op=OR(w725, w724, w723) -> (w722:bool)
    n523 = Compound Arithmetic op=OR(w722, w721, w720) -> (w719:bool)
    n524 = Compound Arithmetic op=OR(w719, w718, w717) -> (w679:bool)
    n525 = Compound Arithmetic op=OR(w679, w544, w543) -> (w670:bool)
    n526 = Compound Arithmetic op=OR(w670, w716, w715) -> (w714:bool)
    n527 = Compound Arithmetic op=OR(w714, w713, w712) -> (w711:bool)
    n528 = Compound Arithmetic op=OR(w711, w710, w709) -> (w708:bool)
    n529 = Compound Arithmetic op=OR(w708, w707, w706) -> (w705:bool)
    n530 = Compound Arithmetic op=OR(w705, w704, w703) -> (w519:bool)
    n531 = Compound Arithmetic op=OR(w519, w547, w546) -> (w528:bool)
    n532 = Compound Arithmetic op=OR(w528, "EXIT HMI", w516) -> (w515:bool)
    "Stop Loops" <- w515
    n533 = property on="Stop Loops" class="Bool (strict)"("Val(Sgnl)"=w515) -> ()  [unwired: 2 in, 2 out]
    n534 = node-c288() -> ()  [unwired: 1 in, 1 out]
  }
  n535 = node-c288(w122) -> (w121:errorcluster)
  n536 = call <userlib>:"Release Writer.vi"("Handle"=w292, "WriteHandle"=w291, "error in (no error)"=w290) -> ("error out"=w298:errorcluster)  [unwired: 11 in, 1 out]
  n537 = call <userlib>:"Release Writer.vi"("Handle"=w272, "WriteHandle"=w271, "error in (no error)"=w270) -> ("error out"=w266:errorcluster)  [unwired: 11 in, 1 out]
  n538 = call <userlib>:"Release Writer.vi"("Handle"=w234, "WriteHandle"=w233, "error in (no error)"=w232) -> ("error out"=w228:errorcluster)  [unwired: 11 in, 1 out]
  n539 = call <userlib>:"Release Type.vi"("Handle"=w287, "TypeHandle"=w288, "error in (no error)"=w289) -> ("error out"=w299:errorcluster)  [unwired: 11 in, 1 out]
  n540 = call <userlib>:"Release Type.vi"("Handle"=w269, "TypeHandle"=w268, "error in (no error)"=w267) -> ("error out"=w265:errorcluster)  [unwired: 11 in, 1 out]
  n541 = call <userlib>:"Release Writer.vi"("Handle"=w253, "WriteHandle"=w252, "error in (no error)"=w251) -> ("error out"=w247:errorcluster)  [unwired: 11 in, 1 out]
  n542 = call <userlib>:"Release Type.vi"("Handle"=w231, "TypeHandle"=w230, "error in (no error)"=w229) -> ("error out"=w227:errorcluster)  [unwired: 11 in, 1 out]
  n543 = call <userlib>:"Release Writer.vi"("Handle"=w215, "WriteHandle"=w214, "error in (no error)"=w213) -> ("error out"=w209:errorcluster)  [unwired: 11 in, 1 out]
  n544 = call <userlib>:"Release Type.vi"("Handle"=w250, "TypeHandle"=w249, "error in (no error)"=w248) -> ("error out"=w246:errorcluster)  [unwired: 11 in, 1 out]
  n545 = call <userlib>:"Release Type.vi"("Handle"=w212, "TypeHandle"=w211, "error in (no error)"=w210) -> ("error out"=w208:errorcluster)  [unwired: 11 in, 1 out]
  n546 = call <userlib>:"Release Writer.vi"("Handle"=w441, "WriteHandle"=w440, "error in (no error)"=w451) -> ("error out"=w141:errorcluster)  [unwired: 11 in, 1 out]
  n547 = call <userlib>:"Release Writer.vi"("Handle"=w310, "WriteHandle"=w309, "error in (no error)"=w308) -> ("error out"=w304:errorcluster)  [unwired: 11 in, 1 out]
  n548 = call <userlib>:"Release Writer.vi"("Handle"=w406, "WriteHandle"=w405, "error in (no error)"=w404) -> ("error out"=w412:errorcluster)  [unwired: 11 in, 1 out]
  n549 = call <userlib>:"Release Writer.vi"("Handle"=w386, "WriteHandle"=w385, "error in (no error)"=w384) -> ("error out"=w380:errorcluster)  [unwired: 11 in, 1 out]
  n550 = call <userlib>:"Release Writer.vi"("Handle"=w348, "WriteHandle"=w347, "error in (no error)"=w346) -> ("error out"=w342:errorcluster)  [unwired: 11 in, 1 out]
  n551 = call <userlib>:"Release Type.vi"("Handle"=w307, "TypeHandle"=w306, "error in (no error)"=w305) -> ("error out"=w303:errorcluster)  [unwired: 11 in, 1 out]
  n552 = call <userlib>:"Release Type.vi"("Handle"=w401, "TypeHandle"=w402, "error in (no error)"=w403) -> ("error out"=w413:errorcluster)  [unwired: 11 in, 1 out]
  n553 = call <userlib>:"Release Type.vi"("Handle"=w383, "TypeHandle"=w382, "error in (no error)"=w381) -> ("error out"=w379:errorcluster)  [unwired: 11 in, 1 out]
  n554 = call <userlib>:"Release Writer.vi"("Handle"=w367, "WriteHandle"=w366, "error in (no error)"=w365) -> ("error out"=w361:errorcluster)  [unwired: 11 in, 1 out]
  n555 = call <userlib>:"Release Type.vi"("Handle"=w345, "TypeHandle"=w344, "error in (no error)"=w343) -> ("error out"=w341:errorcluster)  [unwired: 11 in, 1 out]
  n556 = call <userlib>:"Release Writer.vi"("Handle"=w329, "WriteHandle"=w328, "error in (no error)"=w327) -> ("error out"=w323:errorcluster)  [unwired: 11 in, 1 out]
  n557 = call <userlib>:"Release Type.vi"("Handle"=w364, "TypeHandle"=w363, "error in (no error)"=w362) -> ("error out"=w360:errorcluster)  [unwired: 11 in, 1 out]
  n558 = call <userlib>:"Release Type.vi"("Handle"=w326, "TypeHandle"=w325, "error in (no error)"=w324) -> ("error out"=w322:errorcluster)  [unwired: 11 in, 1 out]
  n559 = call <userlib>:"Release Writer.vi"("Handle"=w424, "WriteHandle"=w423, "error in (no error)"=w422) -> ("error out"=w418:errorcluster)  [unwired: 11 in, 1 out]
  n560 = call <userlib>:"Release Writer.vi"("Handle"=w105, "WriteHandle"=w104, "error in (no error)"=w40) -> ("error out"=w119:errorcluster)  [unwired: 11 in, 1 out]
  n561 = call <userlib>:"Release Writer.vi"("Handle"=w42, "WriteHandle"=w177, "error in (no error)"=w45) -> ("Handle"=w34:u32, "error out"=w183:errorcluster)  [unwired: 11 in]
  n562 = call <userlib>:"Release Type.vi"("Handle"=w421, "TypeHandle"=w420, "error in (no error)"=w419) -> ("error out"=w417:errorcluster)  [unwired: 11 in, 1 out]
  n563 = call <userlib>:"Release Type.vi"("Handle"=w103, "TypeHandle"=w102, "error in (no error)"=w39) -> ("error out"=w118:errorcluster)  [unwired: 11 in, 1 out]
  n564 = call <userlib>:"Release Type.vi"("Handle"=w173, "TypeHandle"=w172, "error in (no error)"=w44) -> ("error out"=w182:errorcluster)  [unwired: 11 in, 1 out]
  n565 = call <userlib>:"Release Type.vi"("Handle"=w439, "TypeHandle"=w438, "error in (no error)"=w450) -> ("error out"=w142:errorcluster)  [unwired: 11 in, 1 out]
  n566 = Merge Errors(w298, w299) -> (w130:errorcluster)
  n567 = Merge Errors(w266, w265) -> (w129:errorcluster)
  n568 = Merge Errors(w228, w227) -> (w127:errorcluster)
  n569 = Merge Errors(w247, w246) -> (w128:errorcluster)
  n570 = Merge Errors(w209, w208) -> (w126:errorcluster)
  n571 = Merge Errors(w412, w413) -> (w136:errorcluster)
  n572 = Merge Errors(w304, w303) -> (w131:errorcluster)
  n573 = Merge Errors(w380, w379) -> (w135:errorcluster)
  n574 = Merge Errors(w342, w341) -> (w133:errorcluster)
  n575 = Merge Errors(w361, w360) -> (w134:errorcluster)
  n576 = Merge Errors(w323, w322) -> (w132:errorcluster)
  n577 = Merge Errors(w418, w417) -> (w137:errorcluster)
  n578 = Merge Errors(w119, w118) -> (w117:errorcluster)
  n579 = Merge Errors(w183, w182) -> (w125:errorcluster)
  n580 = Merge Errors(w141, w142) -> (w140:errorcluster)
  n581 = Merge Errors(w73, w72, w71, w70, w62, w46, w28, w27, w18, w2, w1) -> (w68:errorcluster)
  n582 = Merge Errors(w152, w153, w154, w155, w156, w98, w97, w93, w94, w95, w96) -> (w143:errorcluster)
  n583 = Merge Errors(w120, w151, w150, w149, w148, w147, w146, w145, w84, w83, w82, w69, w68) -> (w144:errorcluster)
  n584 = Merge Errors(w143, w144) -> (w51:errorcluster)
  n585 = Merge Errors(w136, w135, w134, w133, w132, w131, w117) -> (w200:errorcluster)
  n586 = Merge Errors(w130, w129, w128, w127, w126, w31, w125, w35, w37, w57, w56, w55, w52, w24, w21, w15, w12, w8) -> (w199:errorcluster)
  n587 = Merge Errors(w121, w140, w137, w200, w199, w51) -> (w138:errorcluster)
  n588 = call <userlib>:"Release.vi"("Handle"=w34, "error in (no error)"=w138) -> ("error out"=→"error out":errorcluster)  [unwired: 13 in]
